vi "TLB Native Dynamic Events ver 0.17.vi"() -> ()   [LabVIEW 2018]
uses:
  Labview Training Phase 2/Enum Controls/States for Action Engine.ctl
  TLB Type Definitions/State Type Definitions.ctl
  TLB Type Definitions/Intruction Type Definitions.ctl
  TLB Type Definitions/Encoder cluster.ctl
  TLB Type Definitions/PING CLUSTER.ctl
  <vilib>/Studica/Studica Toolkit/NavX/NavX.lvlib
  <vilib>/Studica/Studica Toolkit/Background/DIO Channel.ctl
  Underlying VI's/NavX VI/navX type def.ctl
  <vilib>/myRIO/Instrument Drivers/Utilities/Utilities.lvlib
  <vilib>/Studica/Studica Toolkit/Background/I2C Channel.ctl
  TLB Type Definitions/Vision cluster.ctl
  <vilib>/NI_Real-Time Target Support.lvlib
  TLB Type Definitions/Stepper cluster.ctl
  Experimental VI's/Archived VI's/MOTOR CONTROL NO PID Type Def.ctl
  Underlying VI's/I2C Master VI/I2C MASTER Type Def.ctl
  Underlying VI's/I2C Master VI/I2C_MASTER_WRITE_NEW Type Def.ctl
  <vilib>/userdefined/High Color/IMAQdx.ctl
  Underlying VI's/I2C Master VI/Arduino_Interfacing.ctl
  TLB Type Definitions/Yaw Cluster.ctl
  TLB Type Definitions/Time cluster.ctl
  TLB Type Definitions/Y Stepper cluster.ctl
  Underlying VI's/Modified webcam FGV/Webcam AE.ctl
  Underlying VI's/Elasped Timer/Elapsed timer control.ctl
  Underlying VI's/Motor Control VI with PID/MOTOR CONTROL WITH PID AE DATA MODE TYPE DEF.ctl
  Underlying VI's/Motor Control VI with PID/MOTOR CONTROL WITH PID AE DIRECTION TYPE DEF.ctl
  TLB Type Definitions/IR Sensor Type Def.ctl
  <vilib>/myRIO/Common/Instrument Driver Framework/myRIO v1.0/AI/typedefs/AI Channels Enum.ctl
  <vilib>/myRIO/Common/Instrument Driver Framework/myRIO v1.0/AI/typedefs/AI Channels List.ctl
  <vilib>/Utility/RT CPU Load.ctl
panel:
  out "Left IR Sensor":dbl
  out "Obstacle detected":bool
  out "Speed & distance":T1
  out "Object Center Coordinates":cluster{"x":sgl, "y":sgl}
  out "Object detection cluster":T2
  out "Time up flag":bool
  out "Task selection":u8
  in  "Object recognition mode":enum16{"Ball", "Soap", "Gel", "Pipe", "None"}(ring)
  out "NavX Readings":T3
  out "Arduino Data":T4
  out "CPU loads":T5[](array[typedef]) {"ISR (%)" format="%#.2f"; "Idle (%)" format="%#.2f"; "Background (%)" format="%#.2f"; "Normal (%)" format="%#.2f"; "Above Normal (%)" format="%#.2f"; "High (%)" format="%#.2g"; "Timed Structures (%)" format="%#.2g"; "Time Critical (%)" format="%#.2g"; "Total (%)" format="%#.2g"}
  out "TASK ENABLE":bool
  out "Rising Edge":bool
  in  "Green LED":bool
  out "I2C Error":errorcluster
  out "State Logic":T6=enum."Startup"
  out "elements":T7[](array[typedef])
  in  "STOP TASK":bool
  in  "OK Button":bool
  in  "STOP":bool
  out "error out":errorcluster
  out "Action Queue Items":i32
  out "State Logic Queue Items":i32
  out "Action Queues items":string[](array[string])=["Hardware reset", "Software reset", ""]
  out "Action State":string
  # "System Health Status Update"
  # "VISION"
  # "TLB FRAMEWORK STATUS"
  # "Test Programme written by Calvin Loke    Dated: 28 Aug 2019\nTest Programme revised by Dr Alex See   Dated 30 Aug 2019\n\nRevision date: 20/03/2020\nProgramme version:   TLB Native Dynamic Events ver 0.14a"
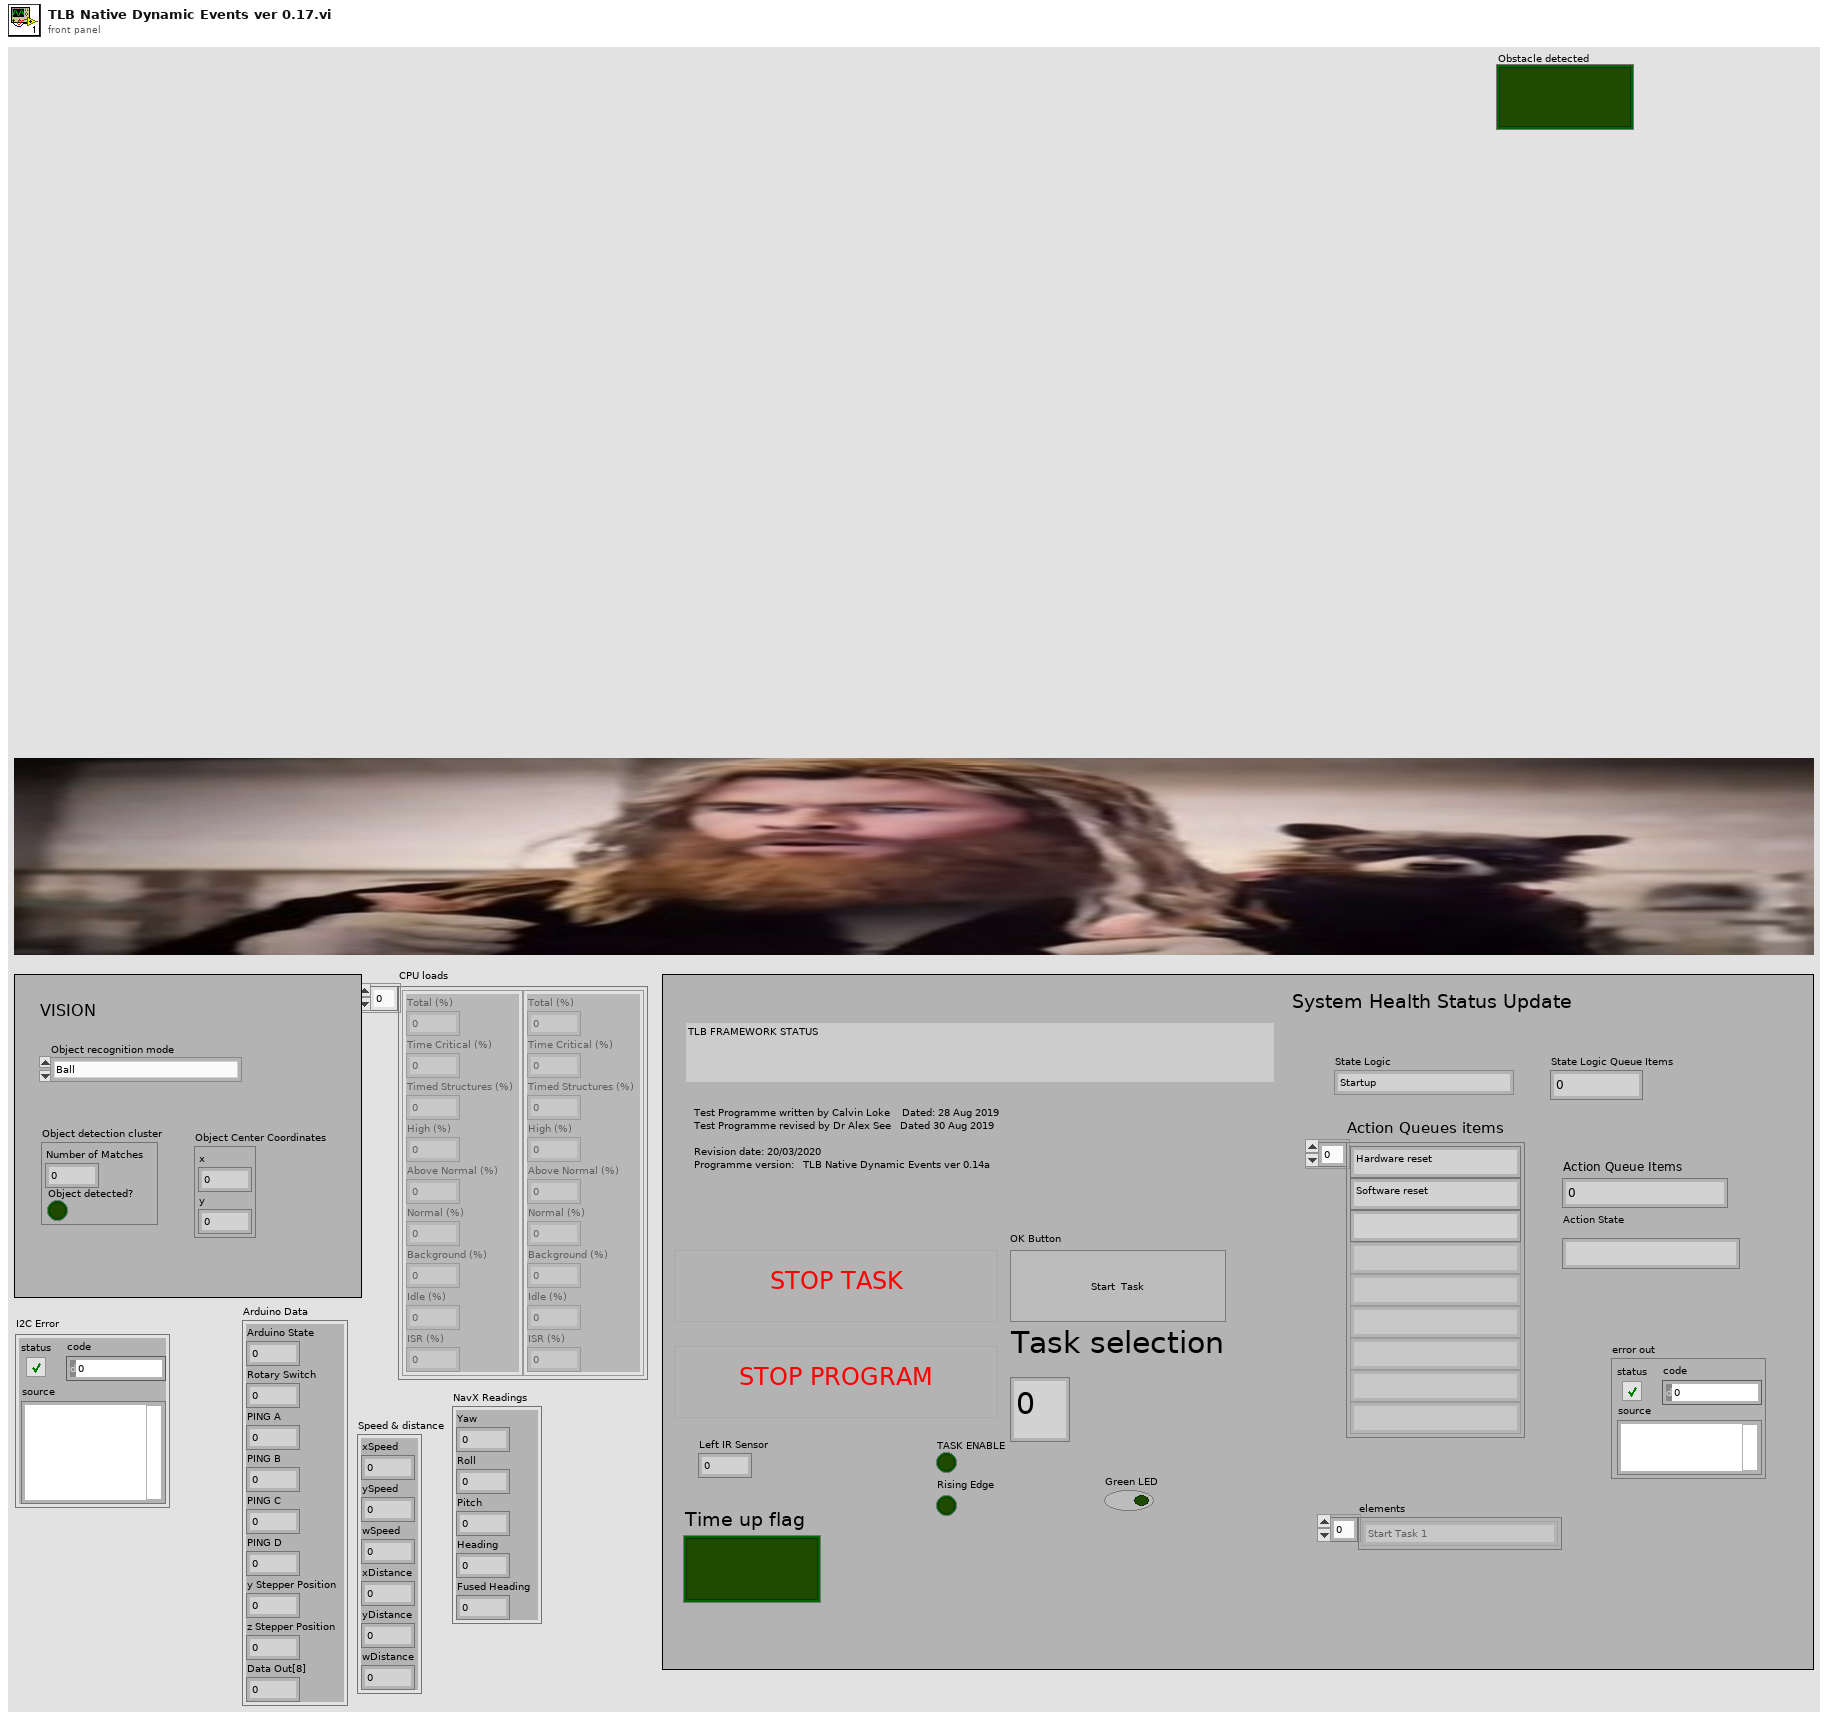
[diagram p1: front panel]
types:
  T1 = cluster{"xSpeed":dbl, "ySpeed":dbl, "wSpeed":dbl, "xDistance":dbl, "yDistance":dbl, "wDistance":dbl}
  T2 = cluster{"Number of Matches":i32, "Object detected?":bool}
  T3 = cluster{"Yaw":dbl, "Roll":dbl, "Pitch":dbl, "Heading":dbl, "Fused Heading":dbl}
  T4 = cluster{"Arduino State":u8, "Rotary Switch":u8, "PING A":u8, "PING B":u8, "PING C":u8, "PING D":u8, "y Stepper Position":u8, "z Stepper Position":u8, "Data Out[8]":u8}
  T5 = typedef "NI_Real-Time Target Support.lvlib/RT CPU Load.ctl" = cluster{"Total (%)":dbl, "Time Critical (%)":dbl, "Timed Structures (%)":dbl, "High (%)":dbl, "Above Normal (%)":dbl, "Normal (%)":dbl, "Background (%)":dbl, "Idle (%)":dbl, "ISR (%)":dbl}
  T6 = typedef "State Type Definitions.ctl" = enum16{"None", "Startup", "Move to Angle", "True Stop", "Idle", "Shutdown", "Task 1A", "Task 1B", "Task 2:Raise Arm", "Task 2:Sensor Mode", "Task 2:Reverse Mode", "Task 3", "Task 4_A", "Task 4_B", "Task 4_C", "Task 4_D", "Task 5A", "Task 5B", "Task 5C", "Task 5D", "Task 5E: POSITION ARM", "Task 5F: ARM GRAB HEIGHT", "Task 5G: CLOSE CLAW", "Task 5H: RAISE ARM", "Task 6_A", "Task 6_B", "Task 7", "Task 8A: RAISE ARM", "Task 8B: MOVE TO BOX", "Task 8C: CAM BURST", "Task 8D: PROCESS IMAGE", "Task 8E: ROBOT ADJUST", "Task 8F: CAM BURST 2", "Task 8G: PROCESS IMAGE 2", "Task 8H: ARM ADJUST", "Task 8I: ARM GRAB HEIGHT", "Task 8J: CLOSE CLAW", "Task 8K: RAISE MY SWORD", "Task 9A: Raise Arm", "Task 9B: Rotate to Angle", "Task 9C: Detect Box", "Task 9D: MOVE FORWARD", "Task 9E: MOVE LEFT", "Task 9F: SCAN IMAGE", "Task 9G: PROCESS COLOUR", "Task 9H: MOVE RIGHT", "Task 9I: SCAN IMAGE", "Task 9J: PROCESS COLOUR", "Task 9K: ROTATE 90 CW", "Task 9L: MOVE FORWARD", "Task 9M: MOVE RIGHT", "Task 9N: SCAN IMAGE", "Task 9O: PROCESS COLOUR", "Task 9P: MOVE RIGHT", "Task 9Q: SCAN IMAGE", "Task 9R: PROCESS COLOUR", "Task A1: Raise Arm", "Task A2: Rotate to Angle", "Task A3: Move Forward", "Task A4: Rotate CW 90"}
  T7 = typedef "Intruction Type Definitions.ctl" = enum16{"None", "Start Task 1", "Start Task 2", "Start Task 3", "Start Task 4", "Start Task 5", "Start Task 6", "Start Task 7", "Start Task 8 - BALL", "Start Task 8 - Gel", "Start Task 8 - Pipe", "Start Task 8 - Soap", "Start Task 9", "Start Task A", "Start Task B", "Exit"}
  T8 = typedef "IR Sensor Type Def.ctl" = cluster{"Left IR Sensor":dbl, "Arm IR Sensor":dbl, "Bottom IR Sensor":dbl}
  T9 = typedef "Y Stepper cluster.ctl" = cluster{"yStepper desired":u8}
  T10 = typedef "Time cluster.ctl" = cluster{"Time up flag":bool, "SET TIME TO CHECK":dbl}
  T11 = typedef "Yaw Cluster.ctl" = cluster{"Yaw":dbl, "Compass":dbl}
  T12 = typedef "Stepper cluster.ctl" = cluster{"y Stepper Position":u8, "z Stepper Position":u8}
  T13 = typedef "DIO Channel.ctl" = enum16{"Not Connected", "A/DIO1", "A/DIO2", "A/DIO3", "A/DIO4", "A/DIO5", "A/DIO6", "A/DIO7", "A/DIO13", "B/DIO1", "B/DIO2", "B/DIO3", "B/DIO4", "B/DIO5", "B/DIO6", "B/DIO7", "B/DIO13", "C/DIO0", "C/DIO1", "C/DIO2", "C/DIO3", "C/DIO4", "C/DIO5", "C/DIO6", "C/DIO7"}
  T14 = typedef "Vision cluster.ctl" = cluster{"Recognized Object":bool, "Object X coordinate":dbl, "Object Y coordinate":dbl}
  T15 = typedef "PING CLUSTER.ctl" = cluster{"PING_A":u8, "PING_B":u8, "PING_C":u8, "PING_D":u8}
  T16 = typedef "Encoder cluster.ctl" = cluster{"xDistance":dbl, "yDistance":dbl, "wDistance":dbl}
  T17 = cluster{"DIO Channel":T13, "FPGA VI Reference Out":refnum<k20>}
  T18 = typedef "navX type def.ctl" = enum16{"Get i2C reference", "Read Values", "Zero Yaw"}
  T19 = typedef "Arduino_Interfacing.ctl" = enum16{"Initialize", "Write to Arduino", "Read From Arduino"}
  T20 = typedef "I2C Channel.ctl" = enum16{"Not Connected", "A", "B"}
  T21 = typedef "States for Action Engine.ctl" = enum16{"Initialize", "Write", "Read"}
  T22 = cluster{"I2C Ref Out":cluster{"I2C Channel":T20, "FPGA VI Reference Out":refnum<k20>}, "Connected":bool, "Slave Address (7-bit)":u8, "Registry":u8[]}
  T23 = typedef "IMAQ Image.ctl" = refnum<image>
  T24 = typedef "State Type Definitions.ctl" = enum16{"None", "Startup", "Move to Angle", "True Stop", "Idle", "Shutdown", "Task 1", "Task 2:Raise Arm", "Task 2:Sensor Mode", "Task 3", "Task 4_A", "Task 4_B", "Task 4_C", "Task 4_D", "Task 5_A", "Task 5 _B", "Task 5_C", "Task 5_D", "Task 5_D_Error", "Task 5D_Error_Right", "Task 5D_Error_Left", "Task 5_E", "Task 5_F", "Task 5F_Error", "Task 5G", "Task 5H", "Task 5I", "Task 6_A", "Task 6_B", "Task 7", "Task 8", "Task 9A: Raise Arm", "Task 9B: Rotate to Angle", "Task 9C: Rotation alignmnet", "Task B"}
  T25 = typedef "MOTOR CONTROL WITH PID AE DIRECTION TYPE DEF.ctl" = enum16{"y-axis movement", "x-axis movement", "rotation", "stop", "reset encoders"}
  T26 = typedef "MOTOR CONTROL WITH PID AE DATA MODE TYPE DEF.ctl" = enum16{"Init AE", "Write to AE", "Read from AE"}
  T27 = typedef "Elapsed timer control.ctl" = enum16{"Start", "Pause", "Initialize"}
  T28 = typedef "I2C_MASTER_WRITE_NEW Type Def.ctl" = enum16{"Ultrasonic sensors", "Stepper origin", "zStepper 13.3k", "zStepper 13k", "zStepper 12k", "zStepper 11k", "zStepper 10k", "zStepper 9k", "zStepper 8k", "zStepper 7k", "zStepper 6k", "zStepper 5k", "zStepper 4k", "zStepper 3k", "zStepper 2k", "zStepper 1k", "zStepper 900", "zStepper 800", "zStepper 700", "zStepper 600", "zStepper 500", "zStepper 400", "zStepper 300", "zStepper 200", "zStepper 100", "zStepper 0", "yStepper control", "Open Claw", "Close Claw", "Soft Reset"}
  T29 = typedef "Webcam AE.ctl" = enum16{"Initialize Camera", "Open Camera", "Continuous Acquisition", "Close Camera", "Retrieve Image", "Dispose Camera Image Buffer"}
  T30 = typedef "IMAQdx.ctl" = refnum<k21>
  T31 = typedef "Webcam AE.ctl" = enum16{"Initialize Camera", "Open Camera", "Continuous Acquisition", "Close Camera", "Retrieve Image", "Dispose Image Buffers"}
  T32 = typedef "MOTOR CONTROL NO PID Type Def.ctl" = enum16{"Init", "Front Back", "Left Right", "Rotate", "Stop", "Latch"}
  T33 = typedef "AI Channels List.ctl" = T34[]
  T34 = typedef "AI Channels Enum.ctl" = enum16{"Not Connected", "AudioIn/Left", "AudioIn/Right", "C/AI0", "C/AI1", "A/AI0", "A/AI1", "A/AI2", "A/AI3", "A/AI4", "A/AI5", "A/AI6", "A/AI7", "B/AI0", "B/AI1", "B/AI2", "B/AI3", "B/AI4", "B/AI5", "B/AI6", "B/AI7", "AI/AI0", "AI/AI1", "AI/AI2", "AI/AI3", "A/AI0 (DIFF)", "A/AI1 (DIFF)", "A/AI2 (DIFF)", "A/AI3 (DIFF)", "B/AI0 (DIFF)", "B/AI1 (DIFF)", "B/AI2 (DIFF)", "B/AI3 (DIFF)"}
  T35 = typedef "I2C MASTER Type Def.ctl" = enum16{"Last State", "Mode 0", "Mode 1", "Mode 2", "Mode 3", "Mode 4", "Mode 5", "Mode 6", "Mode 7", "Mode 8", "Mode 9", "Mode 10"}
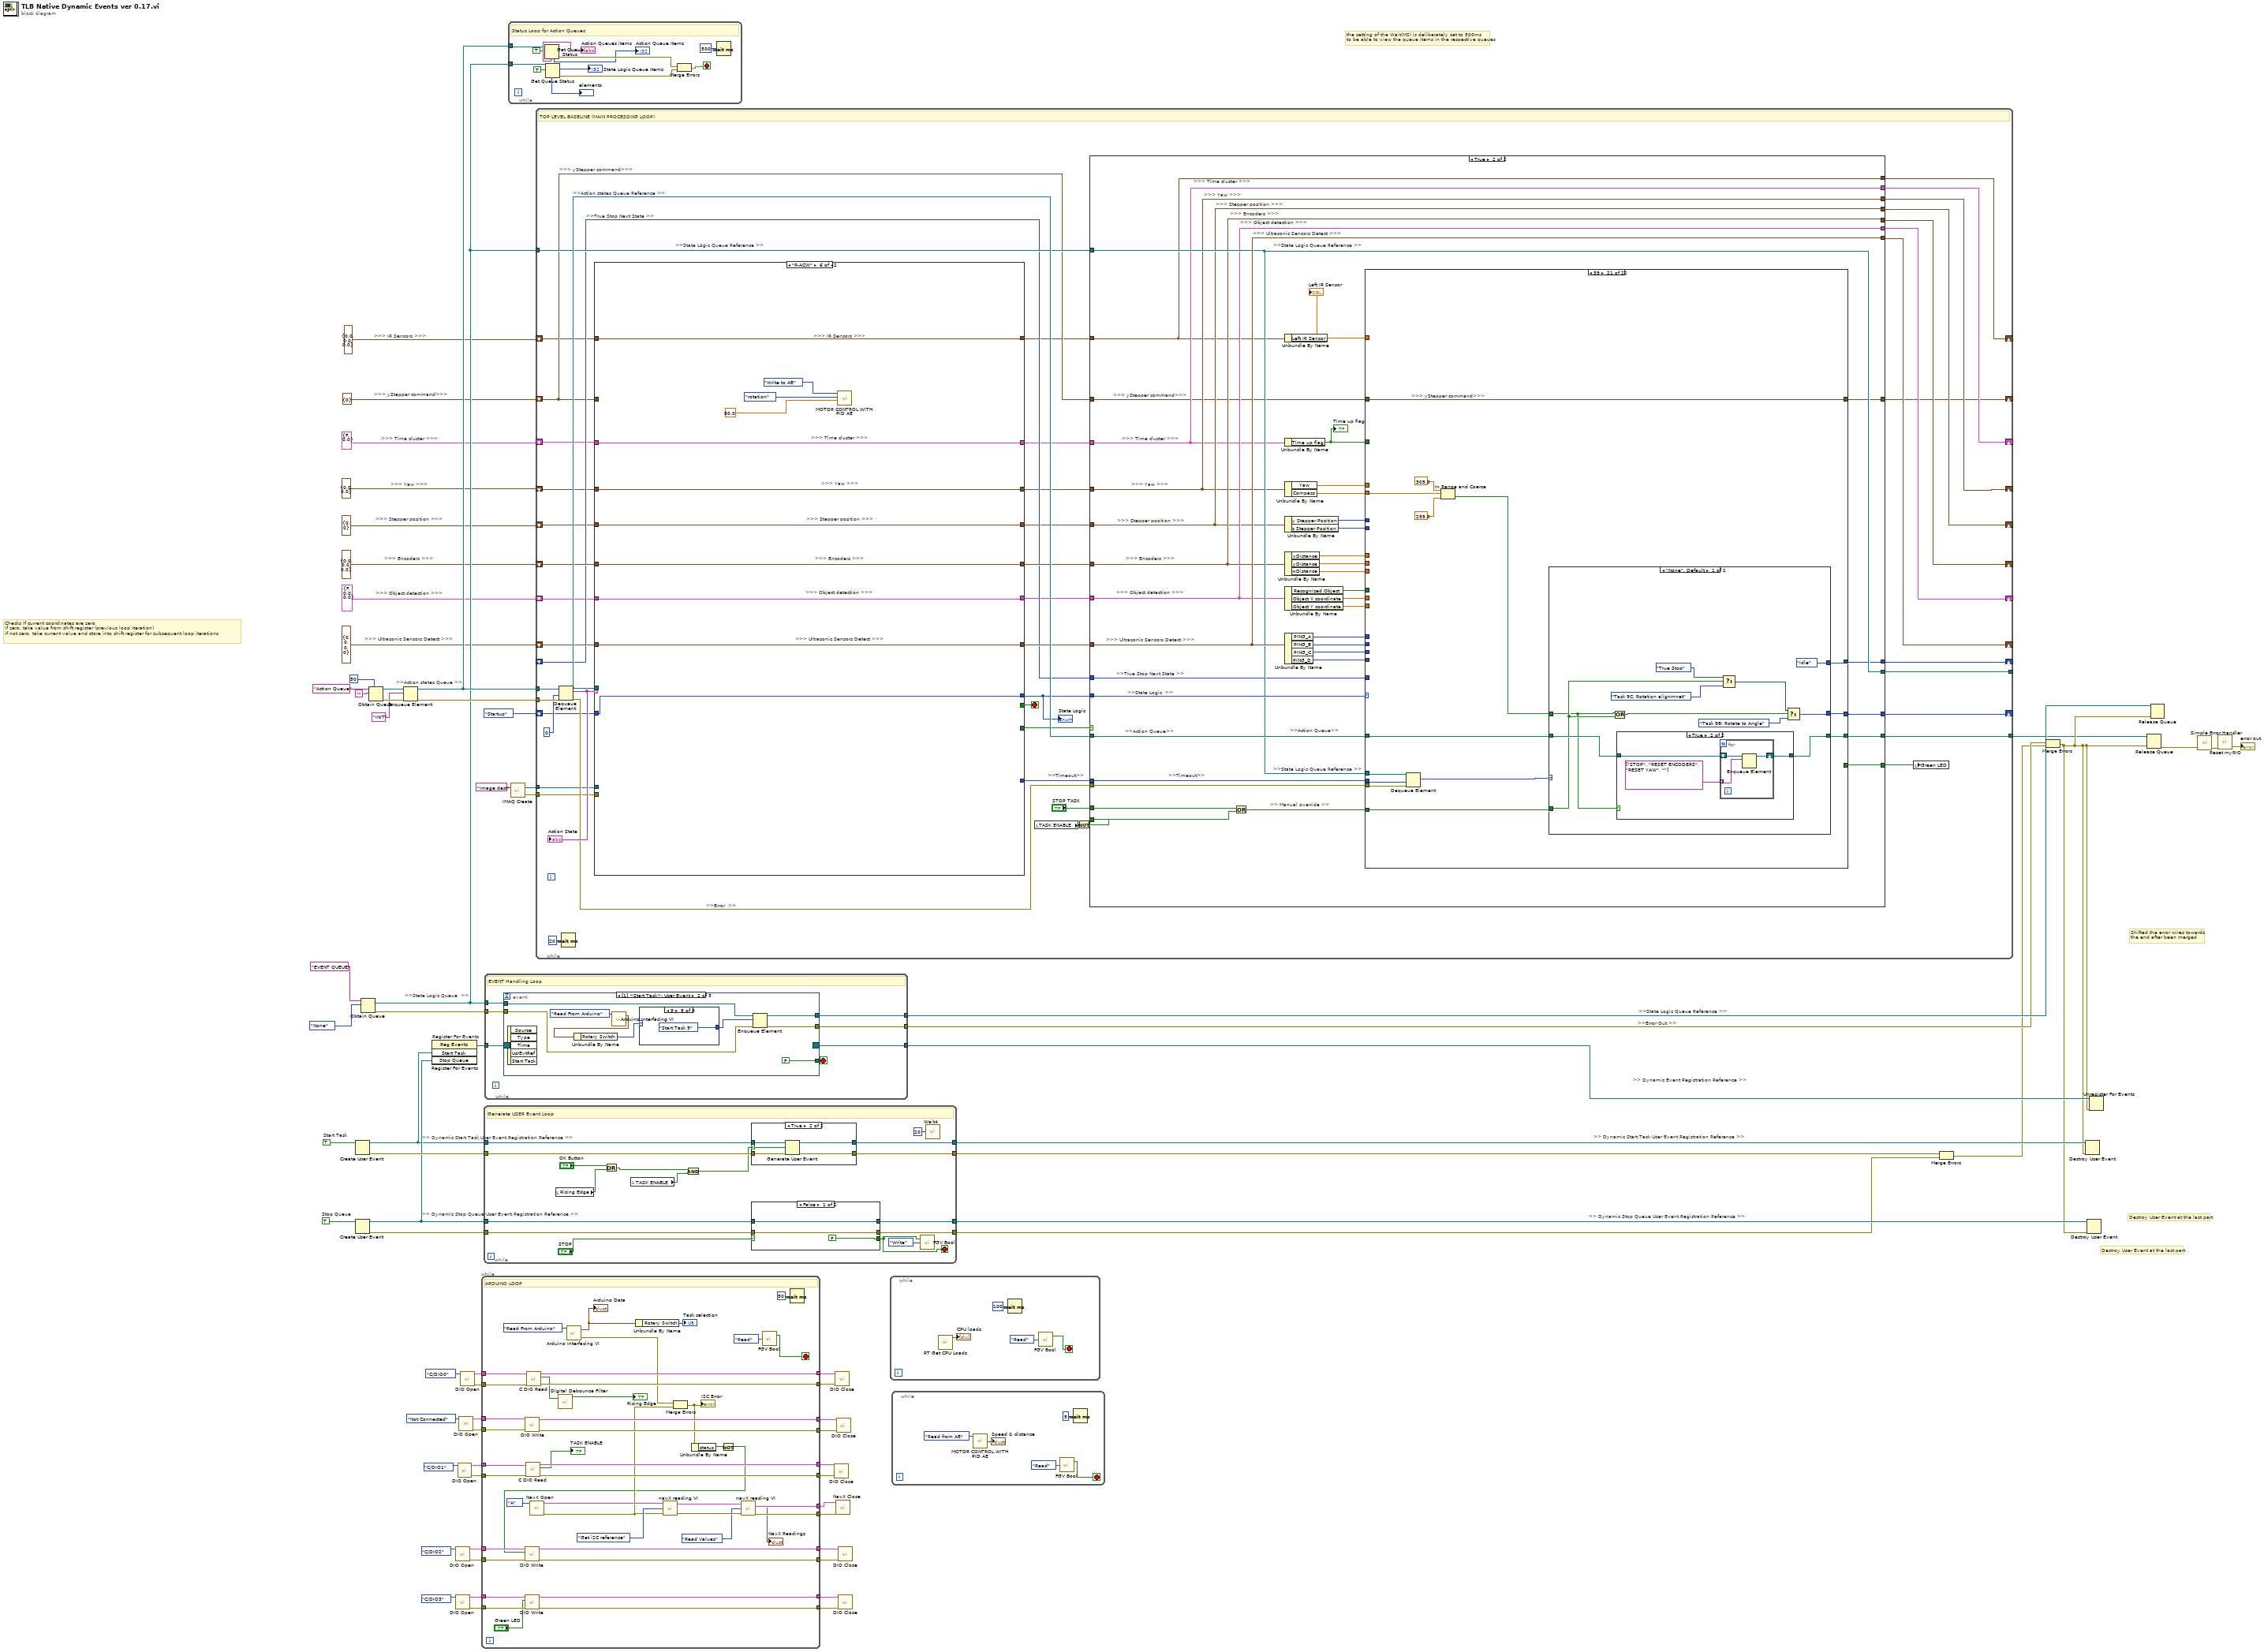
[diagram p0: block diagram]
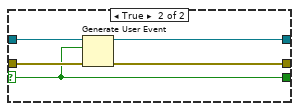
[diagram p2: hidden frame]
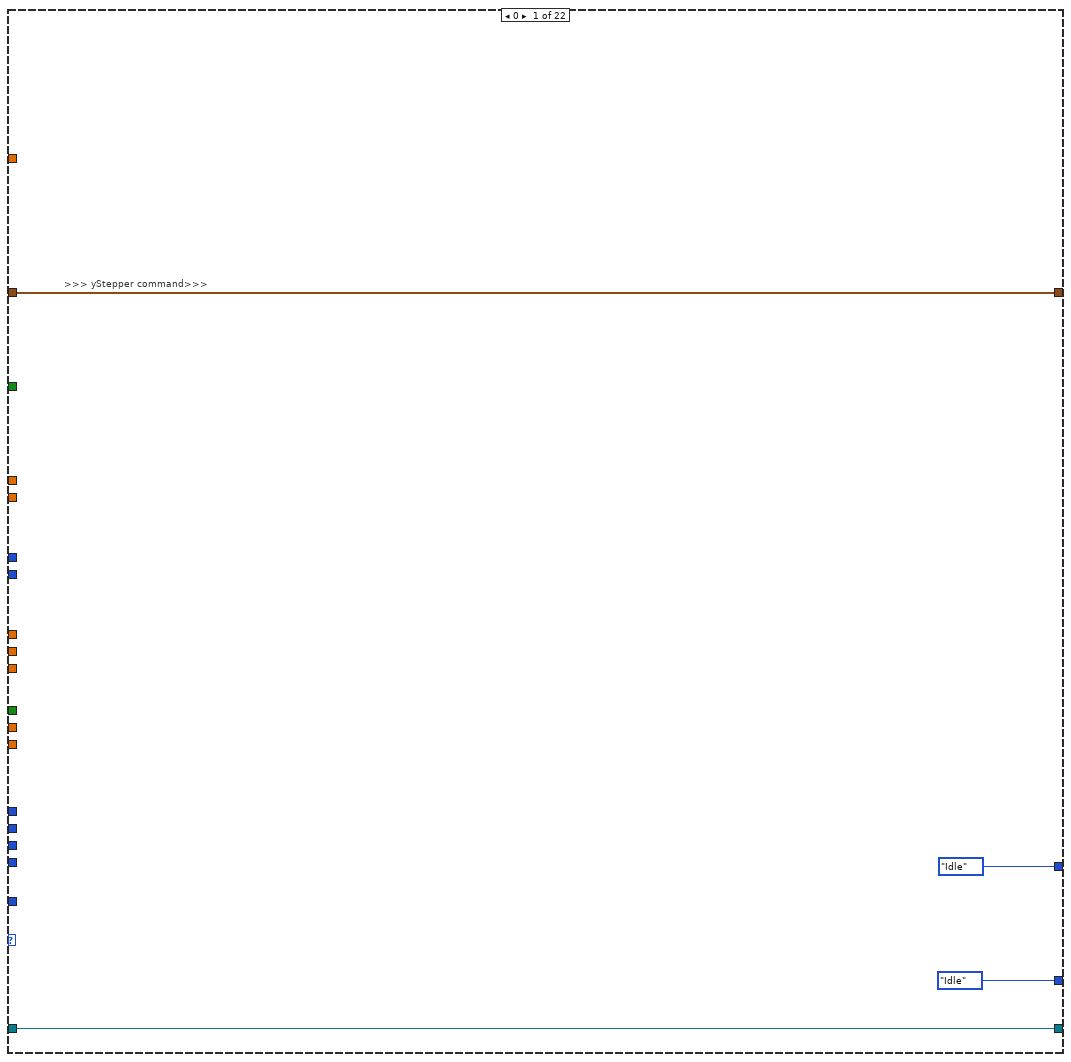
[diagram p5: hidden frame]
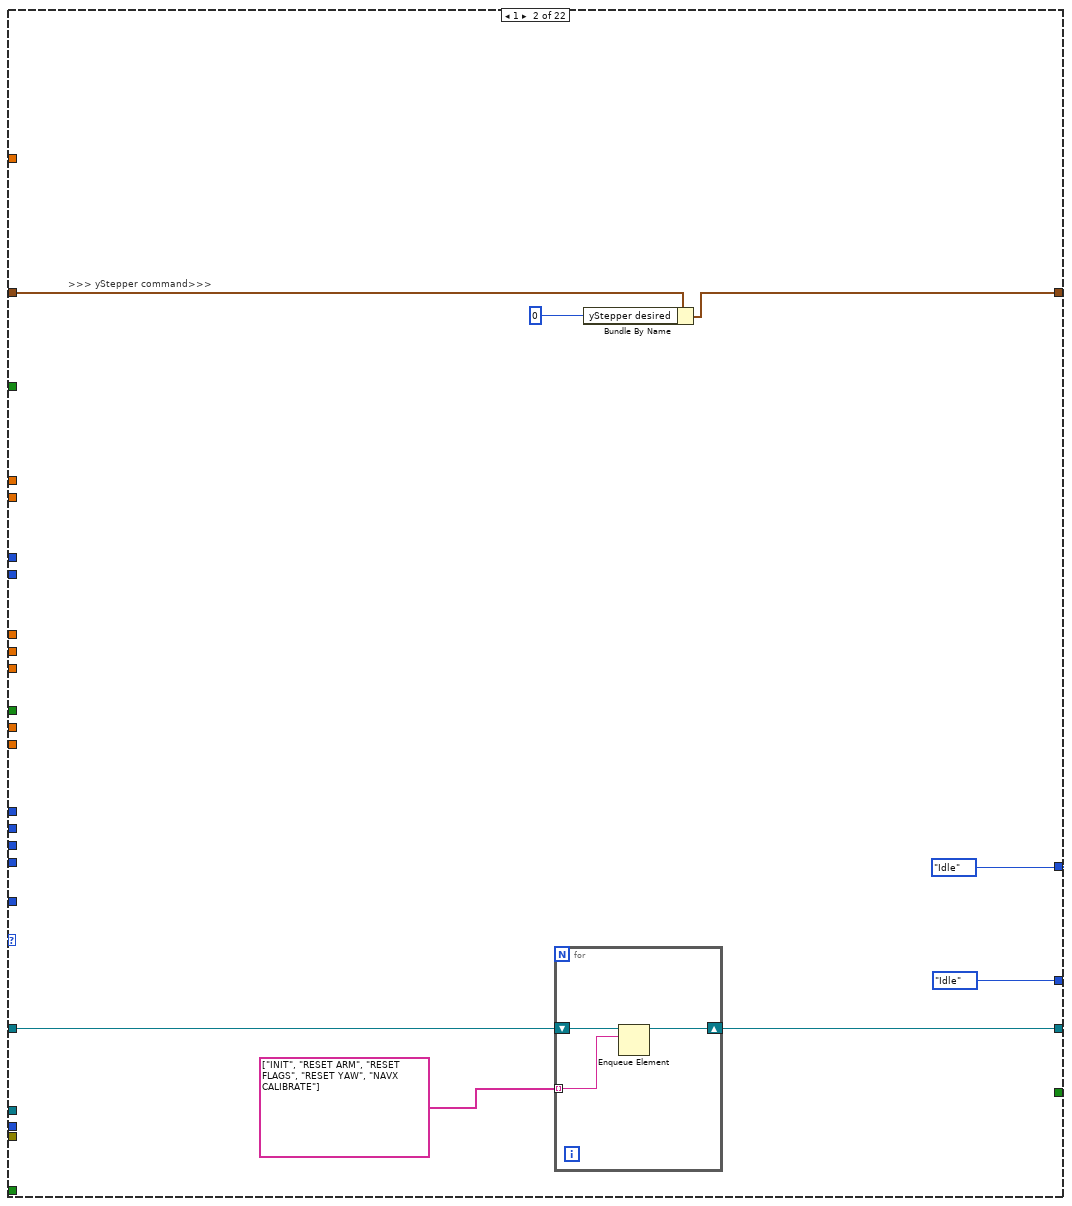
[diagram p6: hidden frame]
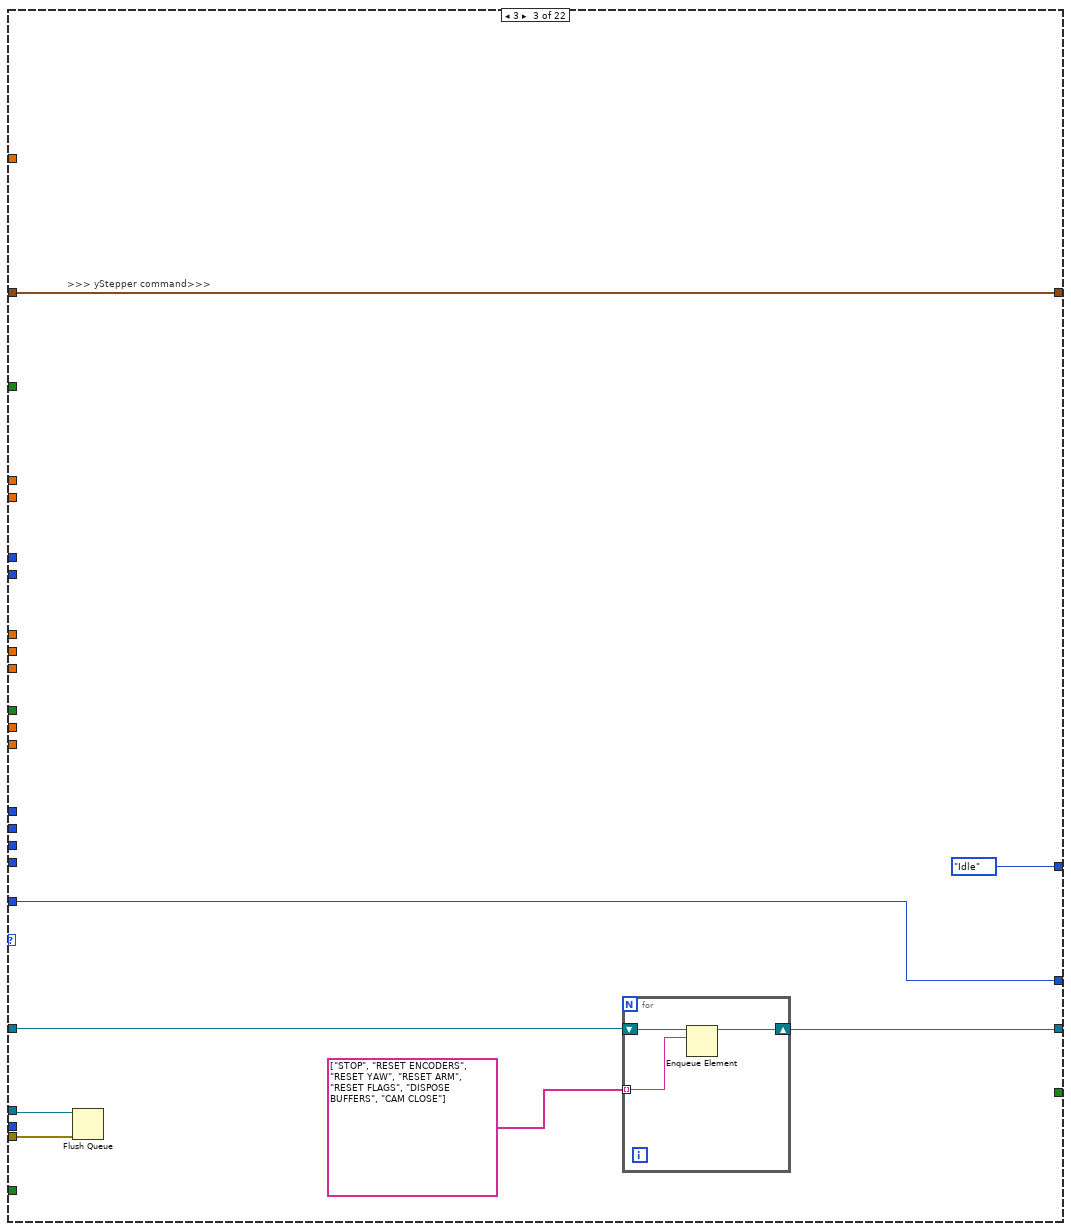
[diagram p7: hidden frame]
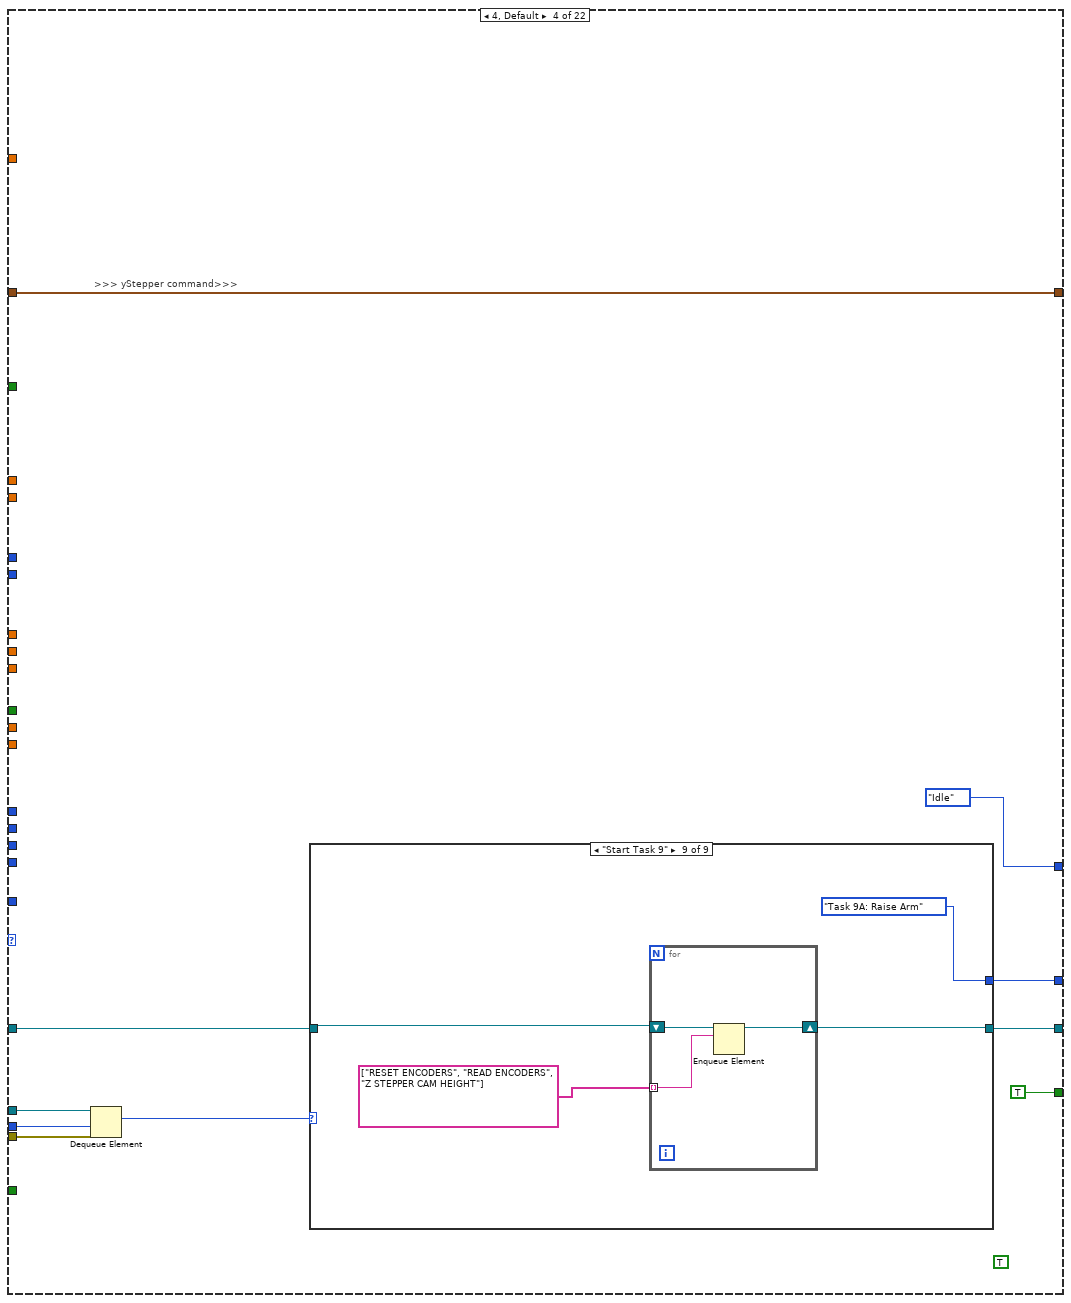
[diagram p8: hidden frame]
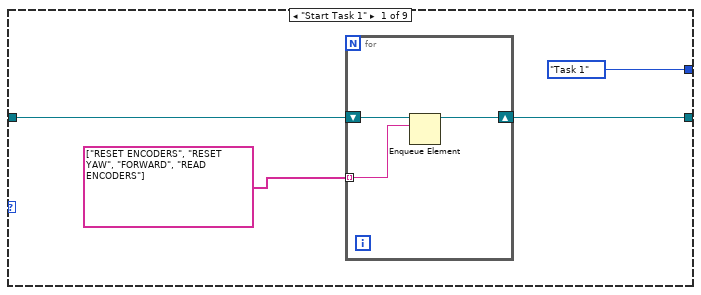
[diagram p9: hidden frame]
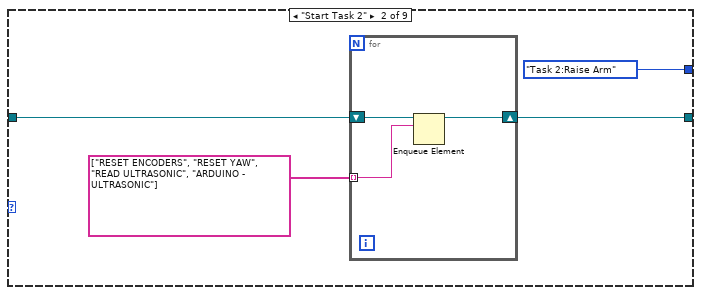
[diagram p10: hidden frame]
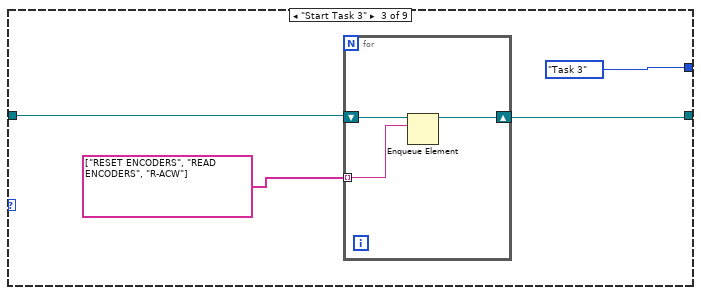
[diagram p11: hidden frame]
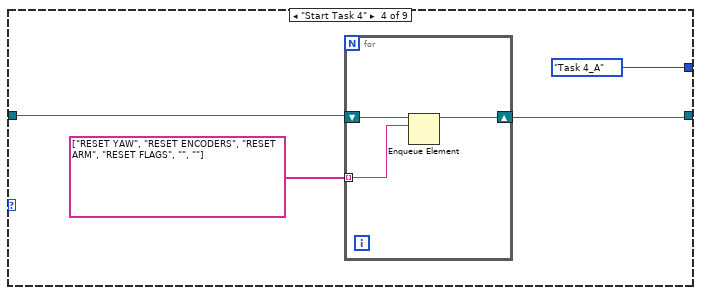
[diagram p12: hidden frame]
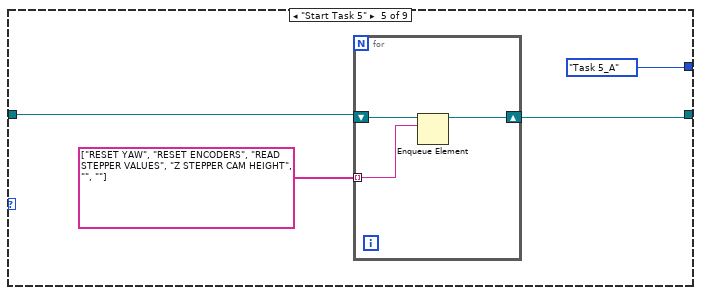
[diagram p13: hidden frame]
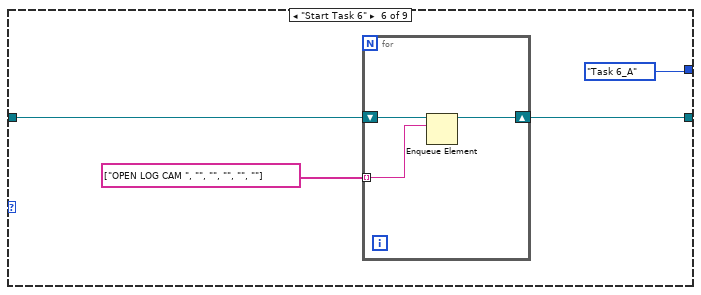
[diagram p14: hidden frame]
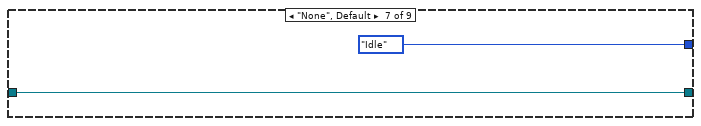
[diagram p15: hidden frame]
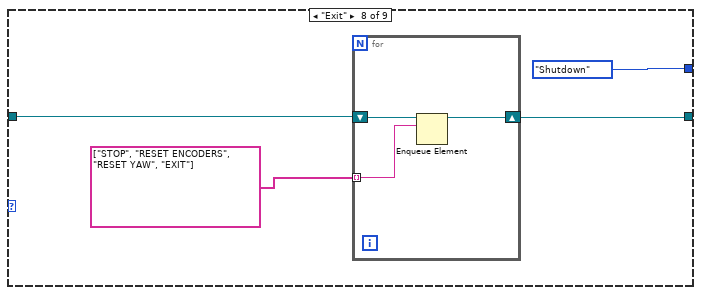
[diagram p16: hidden frame]
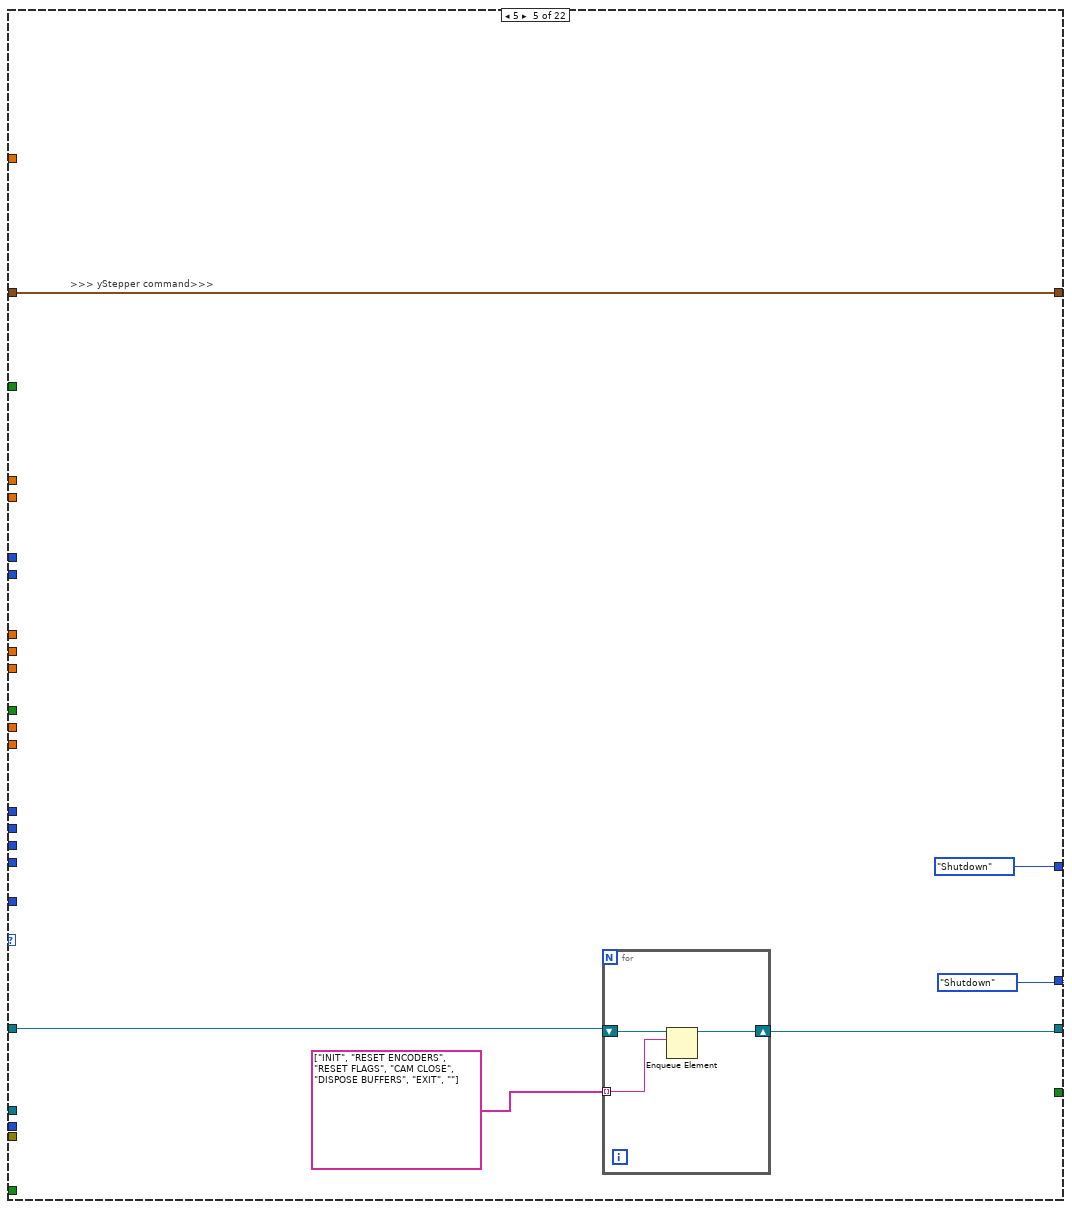
[diagram p17: hidden frame]
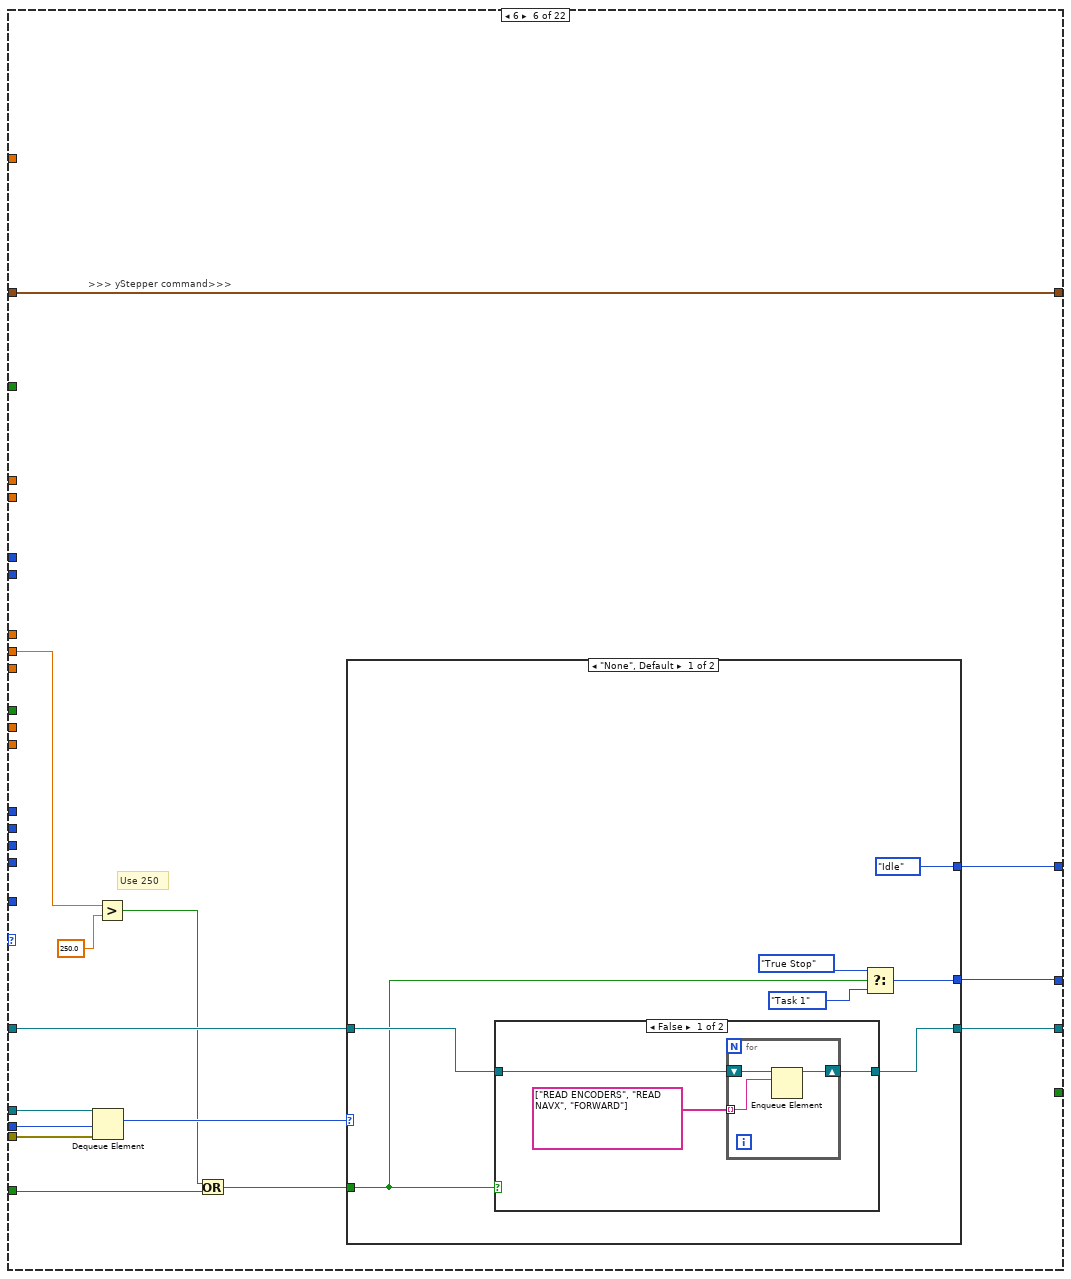
[diagram p18: hidden frame]
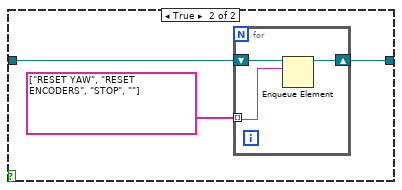
[diagram p19: hidden frame]
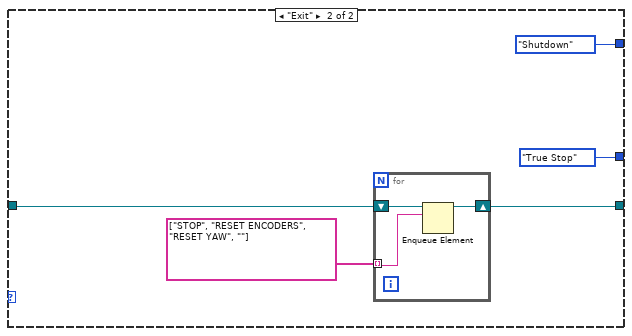
[diagram p20: hidden frame]
diagram:
  w71 = TRUE  # Stop Queue
  w70 = TRUE  # Start Task
  # ">>> IR Sensors >>>"
  # "Checks if current coordinates are zero\nif zero, take value from shift register (previous loop iteration)\nif not zero, take current value and store into shift register for subsequent loop iterations"
  # ">>> yStepper command>>>"
  # ">>> Time cluster >>>"
  # ">>> Yaw >>>"
  # ">>> Stepper position >>>"
  # ">>> Encoders >>>"
  # ">>> Object detection >>>"
  # ">>> Ultrasonic Sensors Detect >>>"
  # "the setting of the Wait(MS) is deliberately set to 500ms\nto be able to view the queue items in the respective queues"
  # ">>Error Out >>"
  # ">> Dynamic Stop Queue User Event Registration Reference >>"
  # ">> Dynamic Start Task User Event Registration Reference >>"
  # ">> Dynamic Stop Queue User Event Registration Reference >>"
  # ">> Dynamic Start Task User Event Registration Reference >>"
  # ">> Dynamic Event Registration Reference >>"
  # ">>Action states Queue >>"
  # ">>State Logic Queue  >>"
  # ">>State Logic Queue Reference >>"
  # "Destroy User Event at the last part"
  # "Destroy User Event at the last part"
  # "Shifted the error wires towards\nthe end after been merged"
  n1 = Create User Event(user event datatype=w70) -> (user event=w62:refnum<user-event>, error out=w67:errorcluster)  [unwired: 1 in]
  n2 = Create User Event(user event datatype=w71) -> (user event=w63:refnum<user-event>, error out=w66:errorcluster)  [unwired: 1 in]
  n3 = Obtain Queue(name (unnamed)="EVENT QUEUE", element data type=Intruction_Type_Definitions."None" ("Enum")) -> (queue out=w48:refnum<queue>, error out=w54:errorcluster)  [unwired: 3 in, 1 out]
  n4 = Obtain Queue(max queue size (-1, unlimited)=50, name (unnamed)="Action Queue", element data type="") -> (queue out=w57:refnum<queue>, error out=w53:errorcluster)  [unwired: 2 in, 1 out]
  n5 = Enqueue Element(queue=w57, element="INIT", error in (no error)=w53) -> (queue out=w49:refnum<queue>, error out=w52:errorcluster)  [unwired: 1 in, 1 out]
  n6 = register-events "Register For Events"(w62, w63) -> (reference out=w61:refnum<event-registration>)  [unwired: 2 in, 1 out]
  n7 = call <vilib>:"DIO Open.vi"("DIO Channel"=DIO_Channel."C/DIO2") -> ("error out"=w15:errorcluster, "DIO Info Out"=w16:T17)  [unwired: 9 in]
  n8 = call <vilib>:"DIO Open.vi"("DIO Channel"=DIO_Channel."C/DIO3") -> ("error out"=w10:errorcluster, "DIO Info Out"=w11:T17)  [unwired: 9 in]
  n9 = call <vilib>:"DIO Open.vi"("DIO Channel"=DIO_Channel."C/DIO1") -> ("error out"=w26:errorcluster, "DIO Info Out"=w27:T17)  [unwired: 9 in]
  n10 = call <vilib>:"DIO Open.vi"("DIO Channel"=DIO_Channel."Not Connected") -> ("error out"=w31:errorcluster, "DIO Info Out"=w33:T17)  [unwired: 9 in]
  n11 = call <vilib>:"DIO Open.vi"("DIO Channel"=DIO_Channel."C/DIO0") -> ("error out"=w36:errorcluster, "DIO Info Out"=w39:T17)  [unwired: 9 in]
  n12 = while {
    tunnel: w39 -> [w112]
    tunnel: [w111] -> w37
    tunnel: w36 -> [w110]
    tunnel: [w109] -> w35
    tunnel: w33 -> [w106]
    tunnel: [w105] -> w32
    tunnel: w31 -> [w104]
    tunnel: [w103] -> w30
    tunnel: [w102] -> w28
    tunnel: w27 -> [w101]
    tunnel: w26 -> [w100]
    tunnel: [w99] -> w25
    tunnel: w16 -> [w93]
    tunnel: w15 -> [w92]
    tunnel: [w91] -> w14
    tunnel: [w90] -> w13
    tunnel: w11 -> [w89]
    tunnel: w10 -> [w88]
    tunnel: [w87] -> w9
    tunnel: [w86] -> w8
    tunnel: [w80] -> w5
    tunnel: [w79] -> w6
    stop <- w114 stop-if-true
    # "ARDUINO LOOP"
    n13 = call <vilib>:"DIO Write.vi"("error in (no error)"=w88, "Input"="Green LED", "DIO Info In"=w89) -> ("error out"=w86:errorcluster, "DIO Info Out"=w87:T17)  [unwired: 7 in]
    n14 = call <vilib>:"DIO Write.vi"("error in (no error)"=w104, "DIO Info In"=w106) -> ("error out"=w103:errorcluster, "DIO Info Out"=w105:T17)  [unwired: 8 in]
    n15 = call <vilib>:"C DIO Read.vi"("error in (no error)"=w100, "DIO Info In in"=w101) -> ("error out"=w99:errorcluster, "IN"=→"TASK ENABLE":bool, "DIO Info In out"=w102:T17)  [unwired: 7 in]
    n16 = call <vilib>:"C DIO Read.vi"("error in (no error)"=w110, "DIO Info In in"=w112) -> ("error out"=w109:errorcluster, "IN"=w108:bool, "DIO Info In out"=w111:T17)  [unwired: 7 in]
    n17 = call <vilib>:"NavX Open.vi"("I2C Channel"=I2C_Channel."A") -> ("error out"=w95:errorcluster, "NavX Info"=w97:T22)  [unwired: 9 in]
    n18 = call "Digital Debounce Filter.vi"("Boolean input"=w108) -> ("Rising Edge"=→"Rising Edge":bool)  [unwired: 1 in, 2 out]
    n19 = call "Arduino Interfacing VI.vi"("AE Mode"=Arduino_Interfacing."Read From Arduino") -> ("error out"=w83:errorcluster, "Arduino Data"=w76:T4)  [unwired: 3 in]
    "Arduino Data" <- w76
    n20 = Unbundle By Name(w76) -> ("Rotary Switch"=→"Task selection":u8)
    n21 = call "navX reading VI.vi"("NavX Info In"=w97, "Mode"=navX_type_def."Get i2C reference", "error in (no error)"=w95) -> ("NavX Info Out"=w82:T22, "Error Out"=w81:errorcluster)  [unwired: 2 out]
    n22 = Merge Errors(w83, w95) -> (w74:errorcluster)
    "I2C Error" <- w74
    n23 = Unbundle By Name(w74) -> ("status"=w73:bool)
    n24 = Not(x=w73) -> (.not. x?=w72:bool)
    n25 = call <vilib>:"DIO Write.vi"("error in (no error)"=w92, "Input"=w72, "DIO Info In"=w93) -> ("error out"=w90:errorcluster, "DIO Info Out"=w91:T17)  [unwired: 7 in]
    n26 = call "navX reading VI.vi"("NavX Info In"=w82, "Mode"=navX_type_def."Read Values", "error in (no error)"=w81) -> ("NavX Info Out"=w80:T22, "NavX Readings"=→"NavX Readings":T3, "Error Out"=w79:errorcluster)  [unwired: 1 out]
    n27 = call "FGV Bool.vi"("Init/Read/Write State"=States_for_Action_Engine."Read") -> ("Output node"=w114:bool)  [unwired: 2 in, 1 out]
    n28 = Wait (ms)(milliseconds to wait=u32 50) -> ()  [unwired: 1 out]
  }
  n29 = while {
    tunnel: w62 -> [w132]
    tunnel: w63 -> [w131]
    tunnel: [w130] -> w69
    tunnel: [w129] -> w68
    tunnel: w67 -> [w128]
    tunnel: [w127] -> w65
    tunnel: w66 -> [w126]
    tunnel: [w125] -> w64
    stop <- w123 stop-if-true
    # "Generate USER Event Loop"
    n30 = local read "Rising Edge"() -> (w119:bool)
    n31 = Or(x="OK Button", y=w119) -> (x .or. y?=w118:bool)
    n32 = local read "TASK ENABLE"() -> (w117:bool)
    n33 = And(x=w118, y=w117) -> (x .and. y?=w116:bool)
    n34 = case shown="True" w116 {
      selector: w116 -> [_ w143]
      tunnel: w132 -> [w142 w147]
      tunnel: [w142 w146] -> w129
      tunnel: w128 -> [w141 w145]
      tunnel: [w141 w144] -> w127
      frame False {
      }
      frame True {
        n35 = Generate User Event(user event=w147, event data cluster=w143, error in=w145) -> (user event out=w146:refnum<user-event>, error out=w144:errorcluster)  [unwired: 1 in]
      }
    }
    n36 = case shown="False" "STOP" {
      selector: "STOP" -> [_ w136]
      tunnel: w131 -> [w135 w140]
      tunnel: [w135 w139] -> w130
      tunnel: w126 -> [w134 w138]
      tunnel: [w134 w137] -> w125
      tunnel: [FALSE w136] -> w123
      frame False {
      }
      frame True {
        n37 = Generate User Event(user event=w140, event data cluster=w136, error in=w138) -> (user event out=w139:refnum<user-event>, error out=w137:errorcluster)  [unwired: 1 in]
      }
    }
    n38 = call "FGV Bool.vi"("Init/Read/Write State"=States_for_Action_Engine."Write", "Input Node"=w123) -> ()  [unwired: 1 in, 2 out]
    n39 = call "Wait4"("Count(uSec)"=u32 20) -> ()  [unwired: 1 out]
  }
  n40 = while {
    tunnel: w61 -> [w154]
    tunnel: [w153] -> w60
    tunnel: w48 -> [w151]
    tunnel: [w150] -> w59
    tunnel: w54 -> [w149]
    tunnel: [w148] -> w51
    stop <- w152 stop-if-true
    # "EVENT Handling Loop"
    n41 = event shown="[1] <Start Task>: User Event" {
      selector: w154 -> [_ _ _]
      dyn-events: [_ _ _] -> w153
      timeout: _ -> [_ _ _]
      tunnel: [FALSE FALSE w183] -> w152
      tunnel: w151 -> [w159 w168 w181]
      tunnel: [w158 w167 w182] -> w150
      tunnel: w149 -> [w157 w166 w180]
      tunnel: [w156 w165 w179] -> w148
      event Timeout {
        n42 = event-data() -> ()  [unwired: 1 in, 3 out]
        n43 = Enqueue Element(queue=w159, element=Intruction_Type_Definitions."None" ("Enum"), error in (no error)=w157) -> (queue out=w158:refnum<queue>, error out=w156:errorcluster)  [unwired: 1 in, 1 out]
      }
      event User Event {
        n44 = event-data() -> ()  [unwired: 1 in, 5 out]
        n45 = call "Arduino Interfacing VI.vi"("AE Mode"=Arduino_Interfacing."Read From Arduino") -> ("Arduino Data"=w162:T4)  [unwired: 3 in, 1 out]
        n46 = Unbundle By Name(w162) -> ("Rotary Switch"=w161:u8)
        n47 = case shown="9" w161 {
          tunnel: [Intruction_Type_Definitions."None" ("Enum") Intruction_Type_Definitions."Start Task 1" ("Enum") Intruction_Type_Definitions."Start Task 2" ("Enum") Intruction_Type_Definitions."Start Task 3" ("Enum") Intruction_Type_Definitions."Start Task 4" ("Enum") Intruction_Type_Definitions."Start Task 5" ("Enum") Intruction_Type_Definitions."Start Task 6" ("Enum") Intruction_Type_Definitions."Start Task 9" ("Enum")] -> w164
          frame 0, Default {
          }
          frame 1 {
          }
          frame 2 {
          }
          frame 3 {
          }
          frame 4 {
          }
          frame 5 {
          }
          frame 6 {
          }
          frame 9 {
          }
        }
        n48 = Enqueue Element(queue=w168, element=w164, error in (no error)=w166) -> (queue out=w167:refnum<queue>, error out=w165:errorcluster)  [unwired: 1 in, 1 out]
      }
      event User Event {
        n49 = event-data() -> ("Stop Queue"=w183:bool)  [unwired: 1 in, 4 out]
        n50 = Enqueue Element At Opposite End(queue=w181, element=Intruction_Type_Definitions."Exit" ("Enum"), error in (no error)=w180) -> (queue out=w182:refnum<queue>, error out=w179:errorcluster)  [unwired: 1 in, 1 out]
      }
    }
  }
  n51 = while {
    tunnel: w49 -> [w193]
    tunnel: w48 -> [w190]
    stop <- w187 stop-if-true
    # "Status Loop for Action Queues"
    n52 = Get Queue Status(queue=w193, return elements? (F)=TRUE) -> (error out=w189:errorcluster, # elements in queue=→"Action Queue Items":i32, elements=→"Action Queues items":string[])  [unwired: 1 in, 5 out]
    n53 = Get Queue Status(queue=w190, return elements? (F)=TRUE) -> (# pending remove=→"State Logic Queue Items":i32, error out=w188:errorcluster, elements=→"elements":T7[])  [unwired: 1 in, 5 out]
    n54 = Merge Errors(w189, w188) -> (w187:errorcluster)
    n55 = Wait (ms)(milliseconds to wait=u32 500) -> ()  [unwired: 1 out]
  }
  n56 = call "IMAQ Create"("Image Name"="Image dest") -> ("New Image"=w20:T23, "error out"=w19:errorcluster)  [unwired: 4 in]
  n57 = while {
    tunnel: w48 -> [w230]
    tunnel: w49 -> [w242]
    tunnel: w52 -> [w240]
    tunnel: [w239] -> _
    tunnel: [w238] -> w42
    shift-right: [w231] -> _
    shift-left: T15 {"PING_A"=0, "PING_B"=0, "PING_C"=0, "PING_D"=0} -> [w233]
    shift-right: [w224] -> _
    shift-left: State_Type_Definitions."Startup" ("Enum") -> [w227]
    shift-right: [w220] -> _
    shift-left: T16 {"xDistance"=0.0, "yDistance"=0.0, "wDistance"=0.0} -> [w222]
    shift-right: [w217] -> _
    shift-left: _ -> [w216]
    tunnel: w20 -> [w215]
    tunnel: w19 -> [w214]
    shift-right: [w211] -> _
    shift-left: T14 {"Recognized Object"=FALSE, "Object X coordinate"=0.0, "Object Y coordinate"=0.0} -> [w213]
    shift-right: [w208] -> _
    shift-left: T12 {"y Stepper Position"=0, "z Stepper Position"=0} -> [w210]
    shift-right: [w205] -> _
    shift-left: T11 {"Yaw"=0.0, "Compass"=0.0} -> [w207]
    shift-right: [w202] -> _
    shift-left: T10 {"Time up flag"=FALSE, "SET TIME TO CHECK"=0.0} -> [w204]
    shift-right: [w200] -> _
    shift-left: T9 {"yStepper desired"=0} -> [w201]
    shift-right: [w196] -> _
    shift-left: T8 {"Left IR Sensor"=0.0, "Arm IR Sensor"=0.0, "Bottom IR Sensor"=0.0} -> [w198]
    stop <- w229 stop-if-true
    # ">>> yStepper command>>>"
    # ">>True Stop Next State >>"
    # ">>Error  >>"
    # ">>Timeout>>"
    # ">>Action states Queue Reference >>"
    # ">>State Logic Queue Reference >>"
    # "TOP LEVEL BASELINE (MAIN PROCESSING LOOP)"
    n58 = Dequeue Element(queue=w242, timeout in ms (-1)=0, error in (no error)=w240) -> (queue out=w234:refnum<queue>, element=w241:string, error out=w235:errorcluster)  [unwired: 1 out]
    "Action State" <- w241
    n59 = Wait (ms)(milliseconds to wait=u32 20) -> ()  [unwired: 1 out]
    n60 = case shown="\"R-ACW\"" w241 {
      tunnel: [_ _ _ _ _ _ _ _ _ _ _ _ _ _ _ _ _ _ 0 w1376 _ _ _ _ _ _ _ _ _ _ _ _ _ _ _ _ _ _ _ _ _ _] -> w237
      tunnel: w234 -> [_ _ _ _ _ _ _ _ _ _ _ _ _ _ _ _ _ _ _ _ _ _ _ _ _ _ _ _ _ _ _ _ _ _ _ _ _ _ _ _ _ _]
      tunnel: w233 -> [w1147 w1156 w1168 w1179 w1196 w1207 w1218 w1230 w1242 w1253 w1260 w1275 w1289 w1301 w1309 w1321 w1346 w1356 w1367 w1377 w1386 w1396 w1426 w1437 w1445 w1454 w1467 w1480 w1490 w1499 w1516 w1525 w1536 w1546 w1556 w1566 w1573 w1585 w1601 w1607 w1619 w1630]
      tunnel: [w1147 w1156 w1168 w1179 w1196 w1207 w1218 w1230 w1242 w1253 w1260 w1275 w1290 w1301 w1309 w1321 w1347 w1356 w1367 w1377 w1386 w1396 w1425 w1437 w1445 w1454 w1467 w1480 w1490 w1499 w1516 w1525 w1536 w1546 w1556 w1566 w1573 w1585 w1601 w1607 w1619 w1630] -> w232
      tunnel: [TRUE TRUE _ _ _ _ _ _ _ _ _ _ _ _ _ _ _ _ _ _ _ _ _ _ _ _ _ _ _ _ _ _ _ _ _ _ _ _ _ _ _ _] -> w229
      tunnel: w227 -> [w1145 w1154 w1167 w1178 w1195 w1206 w1217 w1229 w1241 w1252 w1259 w1274 w1288 w1300 w1307 w1320 w1345 w1355 w1364 w1374 w1385 w1395 w1424 w1436 w1444 w1453 w1466 w1479 w1489 w1498 w1515 w1524 w1535 w1545 w1555 w1565 w1572 w1584 w1600 w1606 w1618 w1629]
      tunnel: [_ _ _ _ _ _ _ _ _ _ _ _ _ _ _ _ _ _ _ TRUE _ _ _ _ _ _ _ _ _ _ _ _ _ _ _ _ _ _ _ _ _ _] -> w226
      tunnel: [w1145 w1154 w1167 w1178 w1195 w1206 w1217 w1229 w1241 w1252 w1259 w1274 w1288 w1300 w1307 w1320 w1345 w1355 w1364 w1374 w1385 w1395 w1424 w1436 w1444 w1453 w1466 w1479 w1489 w1498 w1515 w1524 w1535 w1545 w1555 w1565 w1572 w1584 w1600 w1606 w1618 w1629] -> w225
      tunnel: w222 -> [w1144 w1153 w1166 w1181 w1194 w1205 w1216 w1228 w1240 w1251 w1261 w1273 w1287 w1302 w1311 w1322 w1344 w1357 w1363 w1373 w1387 w1397 w1414 w1435 w1447 w1455 w1468 w1481 w1491 w1500 w1517 w1527 w1538 w1548 w1558 w1568 w1575 w1587 w1603 w1609 w1621 w1632]
      tunnel: [w1144 w1153 w1166 w1181 w1194 w1205 w1216 w1228 w1240 w1251 w1261 w1272 w1287 w1302 w1311 w1322 w1343 w1357 w1363 w1373 w1387 w1397 w1413 w1435 w1447 w1455 w1468 w1481 w1491 w1500 w1517 w1527 w1538 w1548 w1558 w1568 w1575 w1587 w1603 w1609 w1621 w1632] -> w221
      tunnel: w215 -> [w1139 _ _ _ _ _ _ _ _ _ _ _ _ _ _ _ _ _ _ _ _ _ _ _ _ _ _ _ _ _ w1511 _ _ _ _ _ _ _ _ _ _ _]
      tunnel: w214 -> [_ _ _ _ _ _ _ _ _ _ _ _ _ _ _ _ _ _ _ _ _ _ _ _ _ _ _ _ w1483 _ w1513 w1523 _ _ _ _ _ _ _ _ _ _]
      tunnel: w213 -> [w1143 w1152 w1165 w1180 w1193 w1204 w1215 w1227 w1239 w1249 w1258 w1271 w1286 w1295 w1310 w1319 w1335 w1354 w1362 w1372 w1384 w1394 w1419 w1433 w1446 w1452 w1465 w1478 w1485 w1497 w1508 w1526 w1537 w1547 w1557 w1567 w1574 w1586 w1602 w1608 w1620 w1631]
      tunnel: [w1143 w1152 w1165 w1180 w1193 w1204 w1215 w1227 w1239 w1249 w1258 w1271 w1286 w1295 w1310 w1319 w1334 w1354 w1362 w1372 w1384 w1394 w1418 w1433 w1446 w1452 w1465 w1478 w1485 w1497 w1507 w1526 w1537 w1547 w1557 w1567 w1574 w1586 w1602 w1608 w1620 w1631] -> w212
      tunnel: w210 -> [w1142 w1151 w1164 w1182 w1192 w1203 w1214 w1226 w1238 w1248 w1257 w1270 w1285 w1303 w1312 w1318 w1340 w1353 w1361 w1371 w1383 w1393 w1409 w1432 w1443 w1451 w1464 w1477 w1488 w1496 w1518 w1528 w1534 w1544 w1554 w1564 w1576 w1588 w1599 w1610 w1622 w1633]
      tunnel: [w1142 w1151 w1164 w1182 w1192 w1203 w1214 w1226 w1238 w1248 w1257 w1270 w1285 w1303 w1312 w1318 w1339 w1353 w1361 w1371 w1383 w1393 w1408 w1432 w1443 w1451 w1464 w1477 w1488 w1496 w1518 w1528 w1534 w1544 w1554 w1564 w1576 w1588 w1598 w1610 w1622 w1633] -> w209
      tunnel: w207 -> [w1141 w1150 w1162 w1183 w1190 w1201 w1213 w1224 w1236 w1247 w1256 w1269 w1278 w1298 w1313 w1317 w1330 w1352 w1360 w1370 w1382 w1392 w1405 w1431 w1440 w1450 w1463 w1476 w1487 w1495 w1519 w1529 w1533 w1541 w1551 w1561 w1577 w1589 w1593 w1611 w1623 w1634]
      tunnel: [w1141 w1150 w1162 w1183 w1190 w1201 w1213 w1224 w1236 w1247 w1256 w1269 w1278 w1297 w1313 w1317 w1329 w1352 w1360 w1370 w1382 w1392 w1404 w1431 w1440 w1450 w1463 w1476 w1487 w1495 w1519 w1529 w1533 w1541 w1551 w1561 w1577 w1589 w1593 w1611 w1623 w1634] -> w206
      tunnel: w204 -> [w1138 w1149 w1163 w1184 w1191 w1202 w1212 w1225 w1237 w1246 w1255 w1268 w1277 w1294 w1314 w1316 w1326 w1349 w1359 w1369 w1381 w1391 w1402 w1429 w1439 w1449 w1462 w1475 w1486 w1494 w1520 w1530 w1532 w1540 w1550 w1560 w1578 w1590 w1592 w1605 w1617 w1628]
      tunnel: [w1138 w1149 w1163 w1184 w1191 w1202 w1212 w1225 w1237 w1246 w1255 w1268 w1277 w1294 w1314 w1316 w1326 w1349 w1359 w1369 w1381 w1391 w1401 w1429 w1439 w1449 w1462 w1475 w1486 w1494 w1520 w1530 w1532 w1540 w1550 w1560 w1578 w1590 w1592 w1605 w1615 w1627] -> w203
      tunnel: w201 -> [_ _ _ _ _ _ _ _ _ _ _ _ _ _ _ _ _ _ _ _ _ _ _ _ _ _ _ _ _ _ _ _ _ _ _ _ _ w1581 _ _ _ _]
      tunnel: [w1137 w1148 w1157 w1174 w1185 w1197 w1208 w1219 w1231 w1243 w1254 w1262 w1276 w1291 w1305 w1315 w1323 w1348 w1358 w1368 w1380 w1388 w1398 w1428 w1438 w1448 w1456 w1469 w1482 w1492 w1501 w1521 w1531 w1539 w1549 w1559 w1569 w1579 w1591 w1604 w1612 w1624] -> w197
      tunnel: w198 -> [w1137 w1148 w1157 w1174 w1185 w1197 w1208 w1219 w1231 w1243 w1254 w1262 w1276 w1291 w1306 w1315 w1323 w1348 w1358 w1368 w1380 w1388 w1398 w1428 w1438 w1448 w1456 w1469 w1482 w1492 w1501 w1521 w1531 w1539 w1549 w1559 w1569 w1579 w1591 w1604 w1612 w1624]
      frame "Exit" {
        # ">>State Logic  >>"
        # ">>> Time cluster >>>"
        # ">>> Yaw >>>"
        # ">>> Stepper position >>>"
        # ">>> Encoders >>>"
        # ">>> Object detection >>>"
        # ">>> Ultrasonic Sensors Detect >>>"
        n61 = call "Imaq Dispose"("All Images? (No)"=TRUE, "Image"=w1139) -> ()  [unwired: 4 in, 1 out]
      }
      frame "----Movement States----" {
        # ">>State Logic  >>"
        # ">>> Time cluster >>>"
        # ">>> Yaw >>>"
        # ">>> Stepper position >>>"
        # ">>> Encoders >>>"
        # ">>> Object detection >>>"
        # ">>> Ultrasonic Sensors Detect >>>"
      }
      frame "FORWARD" {
        # ">>State Logic  >>"
        # ">>> Time cluster >>>"
        # ">>> Yaw >>>"
        # ">>> Stepper position >>>"
        # ">>> Encoders >>>"
        # ">>> Object detection >>>"
        # ">>> Ultrasonic Sensors Detect >>>"
        n62 = Unbundle By Name(w1162) -> ("Yaw"=w1158:dbl)
        n63 = call "MOTOR CONTROL WITH PID AE.vi"("Yaw"=w1158, "Speed"=50.0, "Direction"=MOTOR_CONTROL_WITH_PID_AE_DIRECTION_TYPE_DEF."y-axis movement", "AE Mode"=MOTOR_CONTROL_WITH_PID_AE_DATA_MODE_TYPE_DEF."Write to AE") -> ()  [unwired: 1 out]
      }
      frame "FORWARD - IR ASSIST" {
        # ">>State Logic  >>"
        # ">>> Time cluster >>>"
        # ">>> Yaw >>>"
        # ">>> Stepper position >>>"
        # ">>> Encoders >>>"
        # ">>> Object detection >>>"
        # ">>> Ultrasonic Sensors Detect >>>"
        n64 = Unbundle By Name(w1174) -> ("Left IR Sensor"=w1173:dbl)
        n65 = Subtract(x=w1173, y=20.0) -> (x-y=w1171:dbl)
        n66 = Multiply(x=w1171, y=0.2) -> (x*y=w1169:dbl)
        n67 = call "MOTOR CONTROL WITH PID AE.vi"("Yaw"=w1169, "Speed"=30.0, "Direction"=MOTOR_CONTROL_WITH_PID_AE_DIRECTION_TYPE_DEF."y-axis movement", "AE Mode"=MOTOR_CONTROL_WITH_PID_AE_DATA_MODE_TYPE_DEF."Write to AE") -> ()  [unwired: 1 out]
      }
      frame "LEFT" {
        # ">>State Logic  >>"
        # ">>> Time cluster >>>"
        # ">>> Yaw >>>"
        # ">>> Stepper position >>>"
        # ">>> Encoders >>>"
        # ">>> Object detection >>>"
        # ">>> Ultrasonic Sensors Detect >>>"
        n68 = Unbundle By Name(w1190) -> ("Yaw"=w1187:dbl)
        n69 = call "MOTOR CONTROL WITH PID AE.vi"("Yaw"=w1187, "Speed"=-25.0, "Direction"=MOTOR_CONTROL_WITH_PID_AE_DIRECTION_TYPE_DEF."x-axis movement", "AE Mode"=MOTOR_CONTROL_WITH_PID_AE_DATA_MODE_TYPE_DEF."Write to AE") -> ()  [unwired: 1 out]
      }
      frame "R-ACW" {
        # ">>> IR Sensors >>>"
        # ">>> Time cluster >>>"
        # ">>> Yaw >>>"
        # ">>> Stepper position >>>"
        # ">>> Encoders >>>"
        # ">>> Object detection >>>"
        # ">>> Ultrasonic Sensors Detect >>>"
        n70 = call "MOTOR CONTROL WITH PID AE.vi"("Speed"=80.0, "Direction"=MOTOR_CONTROL_WITH_PID_AE_DIRECTION_TYPE_DEF."rotation", "AE Mode"=MOTOR_CONTROL_WITH_PID_AE_DATA_MODE_TYPE_DEF."Write to AE") -> ()  [unwired: 1 in, 1 out]
      }
      frame "R-CW" {
        (unwired) -0.2 ("Speed")
        # ">>> Time cluster >>>"
        # ">>> Yaw >>>"
        # ">>> Stepper position >>>"
        # ">>> Encoders >>>"
        # ">>> Object detection >>>"
        # ">>> Ultrasonic Sensors Detect >>>"
        n71 = call "MOTOR CONTROL WITH PID AE.vi"("Speed"=60.0, "Direction"=MOTOR_CONTROL_WITH_PID_AE_DIRECTION_TYPE_DEF."rotation", "AE Mode"=MOTOR_CONTROL_WITH_PID_AE_DATA_MODE_TYPE_DEF."Write to AE") -> ()  [unwired: 1 in, 1 out]
      }
      frame "RIGHT" {
        # ">>> Time cluster >>>"
        # ">>> Yaw >>>"
        # ">>> Stepper position >>>"
        # ">>> Encoders >>>"
        # ">>> Object detection >>>"
        # ">>> Ultrasonic Sensors Detect >>>"
        n72 = Unbundle By Name(w1224) -> ("Yaw"=w1220:dbl)
        n73 = call "MOTOR CONTROL WITH PID AE.vi"("Yaw"=w1220, "Speed"=50.0, "Direction"=MOTOR_CONTROL_WITH_PID_AE_DIRECTION_TYPE_DEF."x-axis movement", "AE Mode"=MOTOR_CONTROL_WITH_PID_AE_DATA_MODE_TYPE_DEF."Write to AE") -> ()  [unwired: 1 out]
      }
      frame "REVERSE" {
        # ">>> Time cluster >>>"
        # ">>> Yaw >>>"
        # ">>> Stepper position >>>"
        # ">>> Encoders >>>"
        # ">>> Object detection >>>"
        # ">>> Ultrasonic Sensors Detect >>>"
        n74 = Unbundle By Name(w1236) -> ("Yaw"=w1232:dbl)
        n75 = call "MOTOR CONTROL WITH PID AE.vi"("Yaw"=w1232, "Speed"=-50.0, "Direction"=MOTOR_CONTROL_WITH_PID_AE_DIRECTION_TYPE_DEF."y-axis movement", "AE Mode"=MOTOR_CONTROL_WITH_PID_AE_DATA_MODE_TYPE_DEF."Write to AE") -> ()  [unwired: 1 out]
      }
      frame "STOP" {
        n76 = Wait (ms)(milliseconds to wait=u32 100) -> ()  [unwired: 1 out]
        n77 = call "MOTOR CONTROL WITH PID AE.vi"("Direction"=MOTOR_CONTROL_WITH_PID_AE_DIRECTION_TYPE_DEF."stop", "AE Mode"=MOTOR_CONTROL_WITH_PID_AE_DATA_MODE_TYPE_DEF."Write to AE") -> ()  [unwired: 2 in, 1 out]
      }
      frame "----SENSOR READING---- " {
      }
      frame "READ ENCODERS" {
        # ">>> Time cluster >>>"
        # ">>> Yaw >>>"
        # ">>> Stepper position >>>"
        # ">>> Object detection >>>"
        # ">>> Current encoder distance >>>"
        # ">>> Ultrasonic Sensors Detect >>>"
        n78 = call "MOTOR CONTROL WITH PID AE.vi"("AE Mode"=MOTOR_CONTROL_WITH_PID_AE_DATA_MODE_TYPE_DEF."Read from AE") -> ("Speed & distance"=w1266:T1)  [unwired: 3 in]
        n79 = Unbundle By Name(w1266) -> ("xDistance"=w1265:dbl, "yDistance"=w1264:dbl, "wDistance"=w1263:dbl)
        n80 = Bundle By Name(cluster=w1273, "xDistance"=w1265, "yDistance"=w1264, "wDistance"=w1263) -> (w1272:T16)
      }
      frame "READ ULTRASONIC" {
        (unwired) navX_type_def."Read Values" ("Mode")
        (unwired) MOTOR_CONTROL_NO_PID_Type_Def."Latch" ("Direction")
        # ">>State Logic  >>"
        # ">>> Time cluster >>>"
        # ">>> Ultrasonic Sensors Detect >>>"
        # ">>> Object detection >>>"
        # ">>> Encoders >>>"
        # ">>> Stepper position >>>"
        # ">>> Yaw >>>"
        n81 = call "Arduino Interfacing VI.vi"("AE Mode"=Arduino_Interfacing."Read From Arduino") -> ("Arduino Data"=w1283:T4)  [unwired: 3 in, 1 out]
        n82 = Unbundle By Name(w1283) -> ("PING A"=w1282:u8, "PING B"=w1281:u8, "PING C"=w1280:u8, "PING D"=w1279:u8)
        n83 = Bundle By Name(cluster=w1289, "PING_A"=w1282, "PING_B"=w1281, "PING_C"=w1280, "PING_D"=w1279) -> (w1290:T15)
      }
      frame "READ NAVX" {
        # ">>> Time cluster >>>"
        # ">>> Yaw >>>"
        # ">>> Ultrasonic Sensors Detect >>>"
        # ">>> Object detection >>>"
        # ">>> Encoders >>>"
        # ">>> Stepper position >>>"
        n84 = call "navX reading VI.vi"("Mode"=navX_type_def."Read Values") -> ("NavX Readings"=w1293:T3)  [unwired: 2 in, 3 out]
        n85 = Unbundle By Name(w1293) -> ("Heading"=w1292:dbl)
        n86 = Unbundle By Name(w1293) -> ("Yaw"=w1296:dbl)
        n87 = Bundle By Name(cluster=w1298, "Yaw"=w1296, "Compass"=w1292) -> (w1297:T11)
      }
      frame "READ IR" {
        w1308 = T33 [enum."A/AI0"] items=["Not Connected", "AudioIn/Left", "AudioIn/Right", "C/AI0", "C/AI1", "A/AI0", "A/AI1", "A/AI2", "A/AI3", "A/AI4", "A/AI5", "A/AI6", "A/AI7", "B/AI0", "B/AI1", "B/AI2", "B/AI3", "B/AI4", "B/AI5", "B/AI6", "B/AI7", "AI/AI0", "AI/AI1", "AI/AI2", "AI/AI3", "A/AI0 (DIFF)", "A/AI1 (DIFF)", "A/AI2 (DIFF)", "A/AI3 (DIFF)", "B/AI0 (DIFF)", "B/AI1 (DIFF)", "B/AI2 (DIFF)", "B/AI3 (DIFF)"] ("AI Channel")
        # ">>State Logic  >>"
        # ">>> Time cluster >>>"
        # ">>> Ultrasonic Sensors Detect >>>"
        # ">>> Object detection >>>"
        # ">>> Encoders >>>"
        # ">>> Stepper position >>>"
        # ">>> Yaw >>>"
        n88 = call <vilib>:"Sharp IR.vi"("AI Channel"=w1308) -> ("Sharp IR Distance"=w1304:dbl)  [unwired: 8 in, 2 out]
        n89 = Bundle By Name(cluster=w1306, "Left IR Sensor"=w1304) -> (w1305:T8)
      }
      frame "----SYSTEM MODES----" {
        (unwired) I2C_MASTER_Type_Def."Last State" ("Arduino Mode")
        # ">>> Object detection >>>"
        # ">>> Yaw >>>"
        # ">>> Ultrasonic Sensors Detect >>>"
        # ">>> Encoders >>>"
        # ">>> Stepper position >>>"
      }
      frame "INIT" {
        w1341 = u8 0
        w1342 = 0.0
        # ">>> Time cluster >>>"
        # ">>> Object detection >>>"
        # ">>> Yaw >>>"
        # ">>> Ultrasonic Sensors Detect >>>"
        # ">>> Encoders >>>"
        # ">>> Stepper position >>>"
        # ">>State Logic  >>"
        n90 = call "Arduino Interfacing VI.vi"("AE Mode"=Arduino_Interfacing."Initialize") -> ()  [unwired: 3 in, 2 out]
        n91 = call "FGV Bool.vi"("Init/Read/Write State"=States_for_Action_Engine."Initialize") -> ()  [unwired: 2 in, 2 out]
        n92 = call "Elasped Timer.vi"("Action"=Elapsed_timer_control."Initialize") -> ()  [unwired: 7 in, 4 out]
        n93 = call "MOTOR CONTROL WITH PID AE.vi"("AE Mode"=MOTOR_CONTROL_WITH_PID_AE_DATA_MODE_TYPE_DEF."Init AE") -> ()  [unwired: 3 in, 1 out]
        n94 = Bundle By Name(cluster=w1335, "Recognized Object"=FALSE, "Object X coordinate"=0.0, "Object Y coordinate"=0.0) -> (w1334:T14)
        n95 = Bundle By Name(cluster=w1340, "y Stepper Position"=u8 0, "z Stepper Position"=u8 0) -> (w1339:T12)
        n96 = Bundle By Name(cluster=w1344, "xDistance"=w1342, "yDistance"=w1342, "wDistance"=w1342) -> (w1343:T16)
        n97 = Bundle By Name(cluster=w1346, "PING_A"=w1341, "PING_B"=w1341, "PING_C"=w1341, "PING_D"=w1341) -> (w1347:T15)
        n98 = Bundle By Name(cluster=w1330, "Yaw"=0.0) -> (w1329:T11)
      }
      frame "ARDUINO - ULTRASONIC" {
        # ">>> Object detection >>>"
        # ">>> Yaw >>>"
        # ">>> Ultrasonic Sensors Detect >>>"
        # ">>> Encoders >>>"
        # ">>> Stepper position >>>"
        # ">>State Logic  >>"
        n99 = call "Arduino Interfacing VI.vi"("Data to Write"=I2C_MASTER_WRITE_NEW_Type_Def."Ultrasonic sensors", "AE Mode"=Arduino_Interfacing."Write to Arduino") -> ()  [unwired: 2 in, 2 out]
      }
      frame "NAVX CALIBRATE" {
        # ">>> Object detection >>>"
        # ">>> Yaw >>>"
        # ">>> Ultrasonic Sensors Detect >>>"
        # ">>> Encoders >>>"
        # ">>> Stepper position >>>"
        # ">>State Logic  >>"
        # "Adds a 15 second delay to the startup process \nfor the NavX to calibrate"
        n100 = Wait (ms)(milliseconds to wait=u32 5000) -> ()  [unwired: 1 out]
      }
      frame "NO ACTION", Default {
        (unwired) u8 0 ("y Stepper value")
        (unwired) TRUE ("Latch")
        (unwired) navX_type_def."Read Values" ("Mode")
        (unwired) MOTOR_CONTROL_NO_PID_Type_Def."Latch" ("Direction")
        # ">>> Object detection >>>"
        # ">>> Yaw >>>"
        # ">>> Ultrasonic Sensors Detect >>>"
        # ">>> Encoders >>>"
        # ">>> Stepper position >>>"
        # ">>State Logic  >>"
        n101 = case shown="4" w1374 {
          tunnel: [0 100] -> w1376
          frame 1, Default {
          }
          frame 4 {
          }
        }
      }
      frame "----RESET CASES----" {
        (unwired) I2C_MASTER_Type_Def."Last State" ("Arduino Mode")
        # ">>> Object detection >>>"
        # ">>> Yaw >>>"
        # ">>> Ultrasonic Sensors Detect >>>"
        # ">>> Encoders >>>"
        # ">>> Stepper position >>>"
        # ">>State Logic  >>"
      }
      frame "RESET ENCODERS" {
        # ">>> Object detection >>>"
        # ">>> Yaw >>>"
        # ">>> Ultrasonic Sensors Detect >>>"
        # ">>> Encoders >>>"
        # ">>> Stepper position >>>"
        # ">>State Logic  >>"
        n102 = call "MOTOR CONTROL WITH PID AE.vi"("Direction"=MOTOR_CONTROL_WITH_PID_AE_DIRECTION_TYPE_DEF."reset encoders", "AE Mode"=MOTOR_CONTROL_WITH_PID_AE_DATA_MODE_TYPE_DEF."Write to AE") -> ()  [unwired: 2 in, 1 out]
      }
      frame "RESET FLAGS" {
        (unwired) I2C_MASTER_Type_Def."Last State" ("Arduino Mode")
        # "Resets any software variables\nand/or non-critical states"
        n103 = Wait (ms)(milliseconds to wait=u32 20) -> ()  [unwired: 1 out]
        n104 = Bundle By Name(cluster=w1402, "Time up flag"=FALSE, "SET TIME TO CHECK"=0.0) -> (w1401:T10)
        n105 = Bundle By Name(cluster=w1419, "Recognized Object"=FALSE, "Object X coordinate"=0.0, "Object Y coordinate"=0.0) -> (w1418:T14)
        n106 = Bundle By Name(cluster=w1409, "y Stepper Position"=u8 0, "z Stepper Position"=u8 0) -> (w1408:T12)
        n107 = Bundle By Name(cluster=w1414, "xDistance"=0.0, "yDistance"=0.0, "wDistance"=0.0) -> (w1413:T16)
        n108 = Bundle By Name(cluster=w1426, "PING_A"=u8 0, "PING_B"=u8 0, "PING_C"=u8 0, "PING_D"=u8 0) -> (w1425:T15)
        n109 = Bundle By Name(cluster=w1405, "Yaw"=0.0) -> (w1404:T11)
      }
      frame "RESET YAW" {
        n110 = Wait (ms)(milliseconds to wait=u32 100) -> ()  [unwired: 1 out]
        n111 = call "navX reading VI.vi"("Mode"=navX_type_def."Zero Yaw") -> ()  [unwired: 2 in, 4 out]
      }
      frame "RESET ARM" {
        n112 = call "Arduino Interfacing VI.vi"("Data to Write"=I2C_MASTER_WRITE_NEW_Type_Def."Soft Reset", "AE Mode"=Arduino_Interfacing."Write to Arduino") -> ()  [unwired: 2 in, 2 out]
      }
      frame "--------CAM STATES-------" {
      }
      frame "OPEN LOG CAM" {
        n113 = call "Webcam AE.vi"("Session In"=T30 "cam0", "Camera states"=Webcam_AE."Initialize Camera") -> ("error out"=w1459:errorcluster, "Session Out"=w1458:T30)  [unwired: 1 in, 1 out]
        n114 = call "Webcam AE.vi"("error in (no error)"=w1459, "Session In"=w1458, "Camera states"=Webcam_AE."Open Camera") -> ()  [unwired: 3 out]
      }
      frame "OPEN LIFE CAM" {
        n115 = call "Webcam AE.vi"("Session In"=T30 "cam1", "Camera states"=Webcam_AE."Initialize Camera") -> ("error out"=w1472:errorcluster, "Session Out"=w1471:T30)  [unwired: 1 in, 1 out]
        n116 = call "Webcam AE.vi"("error in (no error)"=w1472, "Session In"=w1471, "Camera states"=Webcam_AE."Open Camera") -> ()  [unwired: 3 out]
      }
      frame "CAM ACQ" {
        # ">>State Logic  >>"
        # ">>> Time cluster >>>"
        # ">>> Yaw >>>"
        # ">>> Stepper position >>>"
        # ">>> Encoders >>>"
        # ">>> Object detection >>>"
        # ">>> Ultrasonic Sensors Detect >>>"
        n117 = call "Webcam AE.vi"("error in (no error)"=w1483, "Camera states"=Webcam_AE."Continuous Acquisition") -> ()  [unwired: 1 in, 3 out]
      }
      frame "CAM CLOSE" {
        # ">>State Logic  >>"
        # ">>> Time cluster >>>"
        # ">>> Yaw >>>"
        # ">>> Stepper position >>>"
        # ">>> Encoders >>>"
        # ">>> Object detection >>>"
        # ">>> Ultrasonic Sensors Detect >>>"
        n118 = call "Webcam AE.vi"("Camera states"=Webcam_AE."Close Camera") -> ()  [unwired: 2 in, 3 out]
      }
      frame "PROCESS IMAGE" {
        # ">>State Logic  >>"
        # ">>> Time cluster >>>"
        # ">>> Yaw >>>"
        # ">>> Stepper position >>>"
        # ">>> Encoders >>>"
        # ">>> Object detection >>>"
        # ">>> Ultrasonic Sensors Detect >>>"
        n119 = call "Webcam AE.vi"("error in (no error)"=w1513, "Camera states"=Webcam_AE."Retrieve Image") -> ("error out"=w1509:errorcluster, "Image Out"=w1512:T23)  [unwired: 1 in, 1 out]
        n120 = call "Object Detection SubVI.vi"("Error In"=w1509, "Mode"="Object recognition mode", "Image Dest"=w1511, "Image in"=w1512) -> ("Object Center Coordinates"=w1506:cluster{"x":sgl, "y":sgl}, "Object detection cluster"=w1502:T2)  [unwired: 2 out]
        "Object detection cluster" <- w1502
        "Object Center Coordinates" <- w1506
        n121 = Unbundle By Name(w1502) -> ("Object detected?"=w1503:bool)
        n122 = Unbundle By Name(w1506) -> ("x"=w1505:sgl, "y"=w1504:sgl)
        n123 = Bundle By Name(cluster=w1508, "Recognized Object"=w1503, "Object X coordinate"=w1505, "Object Y coordinate"=w1504) -> (w1507:T14)
      }
      frame "DISPOSE BUFFERS" {
        # ">>State Logic  >>"
        # ">>> Time cluster >>>"
        # ">>> Yaw >>>"
        # ">>> Stepper position >>>"
        # ">>> Encoders >>>"
        # ">>> Object detection >>>"
        # ">>> Ultrasonic Sensors Detect >>>"
        n124 = call "Webcam AE.vi"("error in (no error)"=w1523, "Camera states"=Webcam_AE."Dispose Image Buffers") -> ()  [unwired: 1 in, 3 out]
      }
      frame "-----ARM ACTIONS-----" {
      }
      frame "CLOSE CLAW" {
        n125 = call "Arduino Interfacing VI.vi"("Data to Write"=I2C_MASTER_WRITE_NEW_Type_Def."Close Claw", "AE Mode"=Arduino_Interfacing."Write to Arduino") -> ()  [unwired: 2 in, 2 out]
      }
      frame "OPEN CLAW" {
        n126 = call "Arduino Interfacing VI.vi"("Data to Write"=I2C_MASTER_WRITE_NEW_Type_Def."Open Claw", "AE Mode"=Arduino_Interfacing."Write to Arduino") -> ()  [unwired: 2 in, 2 out]
      }
      frame "Z STEPPER CAM HEIGHT" {
        n127 = call "Arduino Interfacing VI.vi"("Data to Write"=I2C_MASTER_WRITE_NEW_Type_Def."zStepper 8k", "AE Mode"=Arduino_Interfacing."Write to Arduino") -> ()  [unwired: 2 in, 2 out]
      }
      frame "Z STEPPER GRAB HEIGHT" {
        # ">>State Logic  >>"
        # ">>> Time cluster >>>"
        # ">>> Yaw >>>"
        # ">>> Stepper position >>>"
        # ">>> Encoders >>>"
        # ">>> Object detection >>>"
        # ">>> Ultrasonic Sensors Detect >>>"
        n128 = call "Arduino Interfacing VI.vi"("Data to Write"=I2C_MASTER_WRITE_NEW_Type_Def."zStepper 100", "AE Mode"=Arduino_Interfacing."Write to Arduino") -> ()  [unwired: 2 in, 2 out]
      }
      frame "Y STEPPER CONTROL" {
        # ">>State Logic  >>"
        # ">>> yStepper command>>>"
        # ">>> Time cluster >>>"
        # ">>> Yaw >>>"
        # ">>> Stepper position >>>"
        # ">>> Encoders >>>"
        # ">>> Object detection >>>"
        # ">>> Ultrasonic Sensors Detect >>>"
        n129 = Unbundle By Name(w1581) -> ("yStepper desired"=w1580:u8)
        n130 = call "Arduino Interfacing VI.vi"("y Stepper value"=w1580, "Data to Write"=I2C_MASTER_WRITE_NEW_Type_Def."yStepper control", "AE Mode"=Arduino_Interfacing."Write to Arduino") -> ()  [unwired: 1 in, 2 out]
      }
      frame "READ STEPPER VALUES" {
        # ">>State Logic  >>"
        # ">>> Time cluster >>>"
        # ">>> Yaw >>>"
        # ">>> Stepper position >>>"
        # ">>> Encoders >>>"
        # ">>> Object detection >>>"
        # ">>> Ultrasonic Sensors Detect >>>"
        n131 = call "Arduino Interfacing VI.vi"("AE Mode"=Arduino_Interfacing."Read From Arduino") -> ("Arduino Data"=w1596:T4)  [unwired: 3 in, 1 out]
        n132 = Unbundle By Name(w1596) -> ("y Stepper Position"=w1595:u8, "z Stepper Position"=w1594:u8)
        n133 = Bundle By Name(cluster=w1599, "y Stepper Position"=w1595, "z Stepper Position"=w1594) -> (w1598:T12)
      }
      frame " -----TIMING-----" {
        # ">>State Logic  >>"
        # ">>> Time cluster >>>"
        # ">>> Yaw >>>"
        # ">>> Stepper position >>>"
        # ">>> Encoders >>>"
        # ">>> Object detection >>>"
        # ">>> Ultrasonic Sensors Detect >>>"
      }
      frame "SET TIMER" {
        # ">>State Logic  >>"
        # ">>> Time cluster >>>"
        # ">>> Yaw >>>"
        # ">>> Stepper position >>>"
        # ">>> Encoders >>>"
        # ">>> Object detection >>>"
        # ">>> Ultrasonic Sensors Detect >>>"
        n134 = call "Elasped Timer.vi"("Time Setting"=5.0, "Action"=Elapsed_timer_control."Initialize") -> ()  [unwired: 6 in, 4 out]
        n135 = Bundle By Name(cluster=w1617, "Time up flag"=FALSE) -> (w1615:T10)
      }
      frame "START TIMER" {
        # ">>State Logic  >>"
        # ">>> Time cluster >>>"
        # ">>> Yaw >>>"
        # ">>> Stepper position >>>"
        # ">>> Encoders >>>"
        # ">>> Object detection >>>"
        # ">>> Ultrasonic Sensors Detect >>>"
        n136 = call "Elasped Timer.vi"("Action"=Elapsed_timer_control."Start") -> ("Time Out?!"=w1625:bool)  [unwired: 7 in, 3 out]
        n137 = Bundle By Name(cluster=w1628, "Time up flag"=w1625) -> (w1627:T10)
      }
    }
    "State Logic" <- w225
    n138 = local read "TASK ENABLE"() -> (w219:bool)
    n139 = Not(x=w219) -> (.not. x?=w218:bool)
    n140 = case shown="True" w226 {
      tunnel: w230 -> [w254 w287]
      tunnel: w234 -> [w250 w289]
      tunnel: [w254 w287] -> w239
      tunnel: [w250 w290] -> w238
      tunnel: w235 -> [_ w285]
      tunnel: w237 -> [_ w286]
      tunnel: w232 -> [w253 w292]
      tunnel: [w253 w292] -> w231
      tunnel: "STOP TASK" -> [_ w275]
      tunnel: w225 -> [w252 w291]
      tunnel: [w252 w288] -> w224
      tunnel: w221 -> [w251 w281]
      tunnel: [w251 w281] -> w220
      tunnel: w218 -> [_ w276]
      tunnel: [w249 w273] -> w217
      tunnel: w216 -> [w249 w272]
      tunnel: w212 -> [w248 w269]
      tunnel: [w248 w269] -> w211
      tunnel: w209 -> [w247 w265]
      tunnel: [w247 w265] -> w208
      tunnel: w206 -> [w246 w263]
      tunnel: [w246 w263] -> w205
      tunnel: w203 -> [w245 w261]
      tunnel: [w245 w261] -> w202
      tunnel: w201 -> [w244 w260]
      tunnel: [w244 w259] -> w200
      tunnel: [_ w257] -> w199
      tunnel: w197 -> [w243 w255]
      tunnel: [w243 w255] -> w196
      frame False {
        # ">>> IR Sensors >>>"
        # ">>> IR Sensors >>>"
        # ">>> yStepper command>>>"
        # ">>> Time cluster >>>"
        # ">>> Yaw >>>"
        # ">>> Stepper position >>>"
        # ">>> Encoders >>>"
        # ">>> Object detection >>>"
        # ">>> Ultrasonic Sensors Detect >>>"
        # ">>> Time cluster >>>"
        # ">>> Yaw >>>"
        # ">>> Stepper position >>>"
        # ">>> Encoders >>>"
        # ">>> Object detection >>>"
        # ">>> Ultrasonic Sensors Detect >>>"
      }
      frame True {
        # ">>State Logic Queue Reference >>"
        # ">>Timeout>>"
        # ">>> yStepper command>>>"
        # ">>> Time cluster >>>"
        # ">>> Object detection >>>"
        # ">>> Yaw >>>"
        # ">>> Ultrasonic Sensors Detect >>>"
        # ">>> Encoders >>>"
        # ">>> Stepper position >>>"
        # ">>State Logic  >>"
        # ">>True Stop Next State >>"
        # ">>Action Queue>>"
        # ">> Manual override >>"
        # ">>> Time cluster >>>"
        # ">>> Yaw >>>"
        # ">>> Stepper position >>>"
        # ">>> Encoders >>>"
        # ">>> Object detection >>>"
        # ">>> Ultrasonic Sensors Detect >>>"
        # ">>Action Queue>>"
        # ">>State Logic Queue Reference >>"
        n141 = Or(x=w275, y=w276) -> (x .or. y?=w274:bool)
        n142 = Unbundle By Name(w255) -> ("Left IR Sensor"=w256:dbl)
        "Left IR Sensor" <- w256
        n143 = Unbundle By Name(w261) -> ("Time up flag"=w262:bool)
        "Time up flag" <- w262
        n144 = Unbundle By Name(w263) -> ("Yaw"=w264:dbl, "Compass"=w258:dbl)
        n145 = Unbundle By Name(w265) -> ("y Stepper Position"=w267:u8, "z Stepper Position"=w266:u8)
        n146 = Unbundle By Name(w281) -> ("xDistance"=w278:dbl, "yDistance"=w279:dbl, "wDistance"=w280:dbl)
        n147 = Unbundle By Name(w269) -> ("Recognized Object"=w268:bool, "Object X coordinate"=w271:dbl, "Object Y coordinate"=w270:dbl)
        n148 = Unbundle By Name(w292) -> ("PING_A"=w284:u8, "PING_B"=w283:u8, "PING_C"=w282:u8, "PING_D"=w277:u8)
        n149 = case shown="39" w291 {
          tunnel: [w295 w301 w313 w322 w389 w402 w437 w489 w529 w571 w624 w670 w709 w768 w812 w851 w896 w939 w981 w1011 w1058 w1098] -> w290
          tunnel: w289 -> [w295 w304 w314 w325 w391 w403 w446 w487 w530 w577 w617 w673 w716 w758 w815 w857 w895 w934 w972 w1015 w1065 w1103]
          tunnel: [State_Type_Definitions."Idle" ("Enum") State_Type_Definitions."Idle" ("Enum") w309 w324 State_Type_Definitions."Shutdown" ("Enum") w404 w444 w490 w528 w572 w623 w671 w711 w767 w813 w858 w897 w940 w973 w1012 w1059 w1099] -> w288
          tunnel: w287 -> [_ _ w312 w328 _ w409 w440 w486 w537 w576 w621 w674 w715 w765 w810 w856 w893 w937 w980 w1019 w1064 w1106]
          tunnel: w286 -> [_ _ _ w327 _ w408 w439 w485 w536 w575 w620 w667 w714 w764 w809 w855 w892 w936 w978 w1014 w1063 w1105]
          tunnel: w285 -> [_ _ w311 w323 _ w407 w438 w484 w535 w574 w619 w666 w713 w766 w811 w854 w891 w935 w979 w1018 w1062 w1104]
          tunnel: w274 -> [_ _ _ _ _ w401 w445 w483 w532 w570 w622 w672 w717 w759 w816 w852 w894 w938 w976 w1017 w1057 w1102]
          tunnel: w284 -> [_ _ _ _ _ _ _ _ _ _ _ _ _ _ _ _ _ _ _ _ _ _]
          tunnel: w283 -> [_ _ _ _ _ _ _ w482 _ _ w613 w655 w707 _ w802 _ _ _ _ _ _ _]
          tunnel: w282 -> [_ _ _ _ _ _ _ w481 _ _ w614 w656 w708 _ w803 _ _ _ _ _ _ _]
          tunnel: w280 -> [_ _ _ _ _ _ _ _ w534 _ _ _ _ _ _ _ _ _ _ _ _ _]
          tunnel: w279 -> [_ _ _ _ _ w400 _ _ _ _ _ _ w712 _ _ _ _ _ _ _ _ _]
          tunnel: w278 -> [_ _ _ _ _ _ _ _ _ _ _ w661 _ _ _ _ _ _ _ _ _ _]
          tunnel: w277 -> [_ _ _ _ _ _ _ _ _ _ _ _ _ _ _ _ _ _ _ _ _ _]
          tunnel: [State_Type_Definitions."Idle" ("Enum") State_Type_Definitions."Idle" ("Enum") State_Type_Definitions."Idle" ("Enum") State_Type_Definitions."Idle" ("Enum") State_Type_Definitions."Shutdown" ("Enum") w397 w443 w488 w525 w569 w616 w669 w710 w769 w814 w850 w898 w941 w974 w1013 w1060 w1101] -> w273
          tunnel: w272 -> [_ _ w309 _ _ _ _ _ _ _ _ _ _ _ _ _ _ _ _ _ _ _]
          tunnel: w268 -> [_ _ _ _ _ _ _ _ _ _ _ _ _ _ _ _ w888 _ w975 _ _ _]
          tunnel: w271 -> [_ _ _ _ _ _ _ _ _ _ _ _ _ _ _ _ _ _ _ _ _ _]
          tunnel: w270 -> [_ _ _ _ _ _ _ _ _ _ _ _ _ _ _ _ _ _ _ _ _ _]
          tunnel: w267 -> [_ _ _ _ _ _ _ _ _ _ _ _ _ _ _ _ _ _ _ _ _ _]
          tunnel: w266 -> [_ _ _ _ _ _ w442 _ _ w567 _ _ _ w762 _ _ _ w933 _ w1016 _ _]
          tunnel: w264 -> [_ _ _ _ _ _ _ _ _ _ _ _ _ _ _ _ _ _ _ _ _ _]
          tunnel: w262 -> [_ _ _ _ _ _ _ _ _ _ _ _ _ _ _ w848 _ _ _ _ _ _]
          tunnel: w260 -> [w293 w299 w308 w320 w387 w396 w441 w480 w524 w568 w615 w665 w706 w757 w807 w849 w889 w930 w971 w1010 w1061 w1100]
          tunnel: [w293 w298 w308 w320 w387 w396 w441 w480 w524 w568 w615 w665 w706 w757 w807 w849 w889 w930 w971 w1010 w1061 w1100] -> w259
          tunnel: w258 -> [_ _ _ _ _ _ _ _ _ _ _ _ _ _ _ _ _ _ _ _ w1056 _]
          tunnel: [_ _ _ TRUE _ _ _ _ _ _ _ _ _ _ _ _ _ _ _ _ _ _] -> w257
          tunnel: w256 -> [_ _ _ _ _ _ _ _ _ _ _ _ _ _ _ _ _ _ _ _ _ _]
          frame 0 {
            # ">>> yStepper command>>>"
          }
          frame 1 {
            # ">>> yStepper command>>>"
            n150 = for {
              shift-right: [w307] -> w301
              shift-left: w304 -> [w306]
              tunnel: string[] ["INIT", "RESET ARM", "RESET FLAGS", "RESET YAW", "NAVX CALIBRATE"] -> [w305] mode=indexing
              n151 = Enqueue Element(queue=w306, element=w305) -> (queue out=w307:refnum<queue>)  [unwired: 2 in, 2 out]
            }
            n152 = Bundle By Name(cluster=w299, "yStepper desired"=u8 0) -> (w298:T9)
          }
          frame 3 {
            # ">>> yStepper command>>>"
            n153 = Flush Queue(queue=w312, error in (no error)=w311) -> ()  [unwired: 3 out]
            n154 = for {
              shift-right: [w318] -> w313
              shift-left: w314 -> [w317]
              tunnel: string[] ["STOP", "RESET ENCODERS", "RESET YAW", "RESET ARM", "RESET FLAGS", "DISPOSE BUFFERS", "CAM CLOSE"] -> [w316] mode=indexing
              n155 = Enqueue Element(queue=w317, element=w316) -> (queue out=w318:refnum<queue>)  [unwired: 2 in, 2 out]
            }
          }
          frame 4, Default {
            (unwired) TRUE ("Green LED")
            # ">>> yStepper command>>>"
            n156 = Dequeue Element(queue=w328, timeout in ms (-1)=w327, error in (no error)=w323) -> (element=w326:T7)  [unwired: 3 out]
            n157 = case shown="\"Start Task 9\"" w326 {
              tunnel: [w330 w337 w344 w351 w358 w365 w372 w374 w382] -> w322
              tunnel: w325 -> [w331 w338 w345 w352 w359 w366 w372 w375 w381]
              tunnel: [State_Type_Definitions."Task 1" ("Enum") State_Type_Definitions."Task 2:Raise Arm" ("Enum") State_Type_Definitions."Task 3" ("Enum") State_Type_Definitions."Task 4_A" ("Enum") State_Type_Definitions."Task 5_A" ("Enum") State_Type_Definitions."Task 6_A" ("Enum") State_Type_Definitions."Idle" ("Enum") State_Type_Definitions."Shutdown" ("Enum") State_Type_Definitions."Task 9A: Raise Arm" ("Enum")] -> w324
              frame "Start Task 1" {
                n158 = for {
                  shift-right: [w335] -> w330
                  shift-left: w331 -> [w334]
                  tunnel: string[] ["RESET ENCODERS", "RESET YAW", "FORWARD", "READ ENCODERS"] -> [w333] mode=indexing
                  n159 = Enqueue Element(queue=w334, element=w333) -> (queue out=w335:refnum<queue>)  [unwired: 2 in, 2 out]
                }
              }
              frame "Start Task 2" {
                n160 = for {
                  shift-right: [w342] -> w337
                  shift-left: w338 -> [w341]
                  tunnel: string[] ["RESET ENCODERS", "RESET YAW", "READ ULTRASONIC", "ARDUINO - ULTRASONIC"] -> [w340] mode=indexing
                  n161 = Enqueue Element(queue=w341, element=w340) -> (queue out=w342:refnum<queue>)  [unwired: 2 in, 2 out]
                }
              }
              frame "Start Task 3" {
                n162 = for {
                  shift-right: [w349] -> w344
                  shift-left: w345 -> [w348]
                  tunnel: string[] ["RESET ENCODERS", "READ ENCODERS", "R-ACW"] -> [w347] mode=indexing
                  n163 = Enqueue Element(queue=w348, element=w347) -> (queue out=w349:refnum<queue>)  [unwired: 2 in, 2 out]
                }
              }
              frame "Start Task 4" {
                n164 = for {
                  shift-right: [w356] -> w351
                  shift-left: w352 -> [w355]
                  tunnel: string[] ["RESET YAW", "RESET ENCODERS", "RESET ARM", "RESET FLAGS", "", ""] -> [w354] mode=indexing
                  n165 = Enqueue Element(queue=w355, element=w354) -> (queue out=w356:refnum<queue>)  [unwired: 2 in, 2 out]
                }
              }
              frame "Start Task 5" {
                n166 = for {
                  shift-right: [w363] -> w358
                  shift-left: w359 -> [w362]
                  tunnel: string[] ["RESET YAW", "RESET ENCODERS", "READ STEPPER VALUES", "Z STEPPER CAM HEIGHT", "", ""] -> [w361] mode=indexing
                  n167 = Enqueue Element(queue=w362, element=w361) -> (queue out=w363:refnum<queue>)  [unwired: 2 in, 2 out]
                }
              }
              frame "Start Task 6" {
                n168 = for {
                  shift-right: [w370] -> w365
                  shift-left: w366 -> [w369]
                  tunnel: string[] ["OPEN LOG CAM ", "", "", "", "", ""] -> [w368] mode=indexing
                  n169 = Enqueue Element(queue=w369, element=w368) -> (queue out=w370:refnum<queue>)  [unwired: 2 in, 2 out]
                }
              }
              frame "None", Default {
              }
              frame "Exit" {
                n170 = for {
                  shift-right: [w379] -> w374
                  shift-left: w375 -> [w378]
                  tunnel: string[] ["STOP", "RESET ENCODERS", "RESET YAW", "EXIT"] -> [w377] mode=indexing
                  n171 = Enqueue Element(queue=w378, element=w377) -> (queue out=w379:refnum<queue>)  [unwired: 2 in, 2 out]
                }
              }
              frame "Start Task 9" {
                n172 = for {
                  shift-right: [w386] -> w382
                  shift-left: w381 -> [w385]
                  tunnel: string[] ["RESET ENCODERS", "READ ENCODERS", "Z STEPPER CAM HEIGHT"] -> [w384] mode=indexing
                  n173 = Enqueue Element(queue=w385, element=w384) -> (queue out=w386:refnum<queue>)  [unwired: 2 in, 2 out]
                }
              }
            }
          }
          frame 5 {
            # ">>> yStepper command>>>"
            n174 = for {
              shift-right: [w395] -> w389
              shift-left: w391 -> [w394]
              tunnel: string[] ["INIT", "RESET ENCODERS", "RESET FLAGS", "CAM CLOSE", "DISPOSE BUFFERS", "EXIT", ""] -> [w393] mode=indexing
              n175 = Enqueue Element(queue=w394, element=w393) -> (queue out=w395:refnum<queue>)  [unwired: 2 in, 2 out]
            }
          }
          frame 6 {
            # ">>> yStepper command>>>"
            # "Use 250"
            n176 = Dequeue Element(queue=w409, timeout in ms (-1)=w408, error in (no error)=w407) -> (element=w406:T7)  [unwired: 3 out]
            n177 = Greater?(x=w400, y=250.0) -> (0:w398:bool)
            n178 = Or(x=w398, y=w401) -> (x .or. y?=w405:bool)
            n179 = case shown="\"None\", Default" w406 {
              tunnel: w405 -> [w412 _]
              tunnel: [w416 State_Type_Definitions."True Stop" ("Enum")] -> w404
              tunnel: w403 -> [w413 w431]
              tunnel: [w411 w430] -> w402
              tunnel: [State_Type_Definitions."Idle" ("Enum") State_Type_Definitions."Shutdown" ("Enum")] -> w397
              frame "None", Default {
                n180 = case shown="False" w412 {
                  tunnel: w413 -> [w419 w425]
                  tunnel: [w418 w423] -> w411
                  frame False {
                    n181 = for {
                      shift-right: [w421] -> w418
                      shift-left: w419 -> [w422]
                      tunnel: string[] ["READ ENCODERS", "READ NAVX", "FORWARD"] ("element") -> [w420] mode=indexing
                      n182 = Enqueue Element(queue=w422, element=w420) -> (queue out=w421:refnum<queue>)  [unwired: 2 in, 2 out]
                    }
                  }
                  frame True {
                    n183 = for {
                      shift-right: [w427] -> w423
                      shift-left: w425 -> [w428]
                      tunnel: string[] ["RESET YAW", "RESET ENCODERS", "STOP", ""] -> [w426] mode=indexing
                      n184 = Enqueue Element(queue=w428, element=w426) -> (queue out=w427:refnum<queue>)  [unwired: 2 in, 2 out]
                    }
                  }
                }
                n185 = Select(t=State_Type_Definitions."True Stop" ("Enum"), s=w412, f=State_Type_Definitions."Task 1" ("Enum")) -> (s? t:f=w416:u16)
              }
              frame "Exit" {
                n186 = for {
                  shift-right: [w435] -> w430
                  shift-left: w431 -> [w436]
                  tunnel: string[] ["STOP", "RESET ENCODERS", "RESET YAW", ""] -> [w434] mode=indexing
                  n187 = Enqueue Element(queue=w436, element=w434) -> (queue out=w435:refnum<queue>)  [unwired: 2 in, 2 out]
                }
              }
            }
          }
          frame 8 {
            # ">> Stepper height reeached >>"
            # ">>> yStepper command>>>"
            # ">> Manual override >>"
            n188 = Dequeue Element(queue=w440, timeout in ms (-1)=w439, error in (no error)=w438) -> (element=w449:T7)  [unwired: 3 out]
            n189 = Equal?(x=w442, y=u8 80) -> (x = y?=w447:bool)
            n190 = case shown="\"None\", Default" w449 {
              tunnel: [w460 State_Type_Definitions."True Stop" ("Enum")] -> w444
              tunnel: [w458 w475] -> w437
              tunnel: w446 -> [w457 _]
              tunnel: w445 -> [w451 _]
              tunnel: [State_Type_Definitions."Idle" ("Enum") State_Type_Definitions."Shutdown" ("Enum")] -> w443
              tunnel: w447 -> [w450 _]
              frame "None", Default {
                # ">> WIill proceed to part ii if not manual override >>"
                # ">>If ENABLE or Trigger is set to true>>"
                n191 = Or(x=w450, y=w451) -> (x .or. y?=w452:bool)
                n192 = case shown="True" w450 {
                  tunnel: [w463 w469] -> w458
                  tunnel: w457 -> [w462 w468]
                  frame False {
                    n193 = for {
                      shift-right: [w465] -> w463
                      shift-left: w462 -> [w466]
                      tunnel: string[] ["Z STEPPER CAM HEIGHT", "READ STEPPER VALUES"] ("element") -> [w464] mode=indexing
                      n194 = Enqueue Element(queue=w466, element=w464) -> (queue out=w465:refnum<queue>)  [unwired: 2 in, 2 out]
                    }
                  }
                  frame True {
                    n195 = for {
                      shift-right: [w471] -> w469
                      shift-left: w468 -> [w472]
                      tunnel: string[] ["ARDUINO - ULTRASONIC", "READ ULTRASONIC", "", "", "", ""] -> [w470] mode=indexing
                      n196 = Enqueue Element(queue=w472, element=w470) -> (queue out=w471:refnum<queue>)  [unwired: 2 in, 2 out]
                    }
                  }
                }
                n197 = Select(t=State_Type_Definitions."True Stop" ("Enum"), s=w451, f=State_Type_Definitions."Task 2:Sensor Mode" ("Enum")) -> (s? t:f=w454:T6)
                n198 = Select(t=w454, s=w452, f=State_Type_Definitions."Task 2:Raise Arm" ("Enum")) -> (s? t:f=w460:T6)
              }
              frame "Exit" {
                n199 = for {
                  shift-right: [w478] -> w475
                  shift-left: _ -> [w479]
                  tunnel: string[] ["STOP", "RESET ENCODERS", "RESET YAW", ""] -> [w477] mode=indexing
                  n200 = Enqueue Element(queue=w479, element=w477) -> (queue out=w478:refnum<queue>)  [unwired: 2 in, 2 out]
                }
              }
            }
          }
          frame 9 {
            w494 = u8 30 ("y")
            # ">>> yStepper command>>>"
            # ">>Object detected>>"
            n201 = Dequeue Element(queue=w486, timeout in ms (-1)=w485, error in (no error)=w484) -> (element=w495:T7)  [unwired: 3 out]
            n202 = Less?(x=w482, y=w494) -> (x < y?=w493:bool)
            n203 = Less?(x=w481, y=w494) -> (x < y?=w492:bool)
            n204 = Or(x=w493, y=w492) -> (x .or. y?=w491:bool)
            "Obstacle detected" <- w491
            n205 = case shown="\"None\", Default" w495 {
              tunnel: w491 -> [w499 _]
              tunnel: [w501 State_Type_Definitions."True Stop" ("Enum")] -> w490
              tunnel: w483 -> [w500 _]
              tunnel: w487 -> [w498 w518]
              tunnel: [w497 w519] -> w489
              tunnel: [State_Type_Definitions."Idle" ("Enum") State_Type_Definitions."Shutdown" ("Enum")] -> w488
              frame "None", Default {
                n206 = case shown="False" w499 {
                  tunnel: w498 -> [w505 w512]
                  tunnel: [w506 w511] -> w497
                  frame False {
                    n207 = for {
                      tunnel: string[] ["READ ULTRASONIC", "STOP"] ("element") -> [w507] mode=indexing
                      shift-right: [w509] -> w506
                      shift-left: w505 -> [w508]
                      n208 = Enqueue Element(queue=w508, element=w507) -> (queue out=w509:refnum<queue>)  [unwired: 2 in, 2 out]
                    }
                  }
                  frame True {
                    n209 = for {
                      shift-right: [w514] -> w511
                      shift-left: w512 -> [w515]
                      tunnel: string[] ["REVERSE", "READ ULTRASONIC", "READ NAVX"] -> [w513] mode=indexing
                      n210 = Enqueue Element(queue=w515, element=w513) -> (queue out=w514:refnum<queue>)  [unwired: 2 in, 2 out]
                    }
                  }
                }
                n211 = Select(t=State_Type_Definitions."True Stop" ("Enum"), s=w500, f=State_Type_Definitions."Task 2:Sensor Mode" ("Enum")) -> (s? t:f=w501:T6)
              }
              frame "Exit" {
                n212 = for {
                  shift-right: [w522] -> w519
                  shift-left: w518 -> [w523]
                  tunnel: string[] ["STOP", "RESET ENCODERS", "RESET YAW", "ARDUINO MODE 0"] -> [w521] mode=indexing
                  n213 = Enqueue Element(queue=w523, element=w521) -> (queue out=w522:refnum<queue>)  [unwired: 2 in, 2 out]
                }
              }
            }
          }
          frame 11 {
            # ">>> yStepper command>>>"
            n214 = Dequeue Element(queue=w537, timeout in ms (-1)=w536, error in (no error)=w535) -> (element=w526:T7)  [unwired: 3 out]
            n215 = Greater?(x=w534, y=160.0) -> (0:w531:bool)
            n216 = Or(x=w531, y=w532) -> (x .or. y?=w527:bool)
            n217 = case shown="\"None\", Default" w526 {
              tunnel: w527 -> [w540 _]
              tunnel: [w544 State_Type_Definitions."True Stop" ("Enum")] -> w528
              tunnel: w530 -> [w541 w560]
              tunnel: [w539 w559] -> w529
              tunnel: [State_Type_Definitions."Idle" ("Enum") State_Type_Definitions."Shutdown" ("Enum")] -> w525
              frame "None", Default {
                n218 = case shown="False" w540 {
                  tunnel: w541 -> [w547 w553]
                  tunnel: [w546 w551] -> w539
                  frame False {
                    n219 = for {
                      shift-right: [w549] -> w546
                      shift-left: w547 -> [w550]
                      tunnel: string[] ["READ ENCODERS", "R-ACW"] ("element") -> [w548] mode=indexing
                      n220 = Enqueue Element(queue=w550, element=w548) -> (queue out=w549:refnum<queue>)  [unwired: 2 in, 2 out]
                    }
                  }
                  frame True {
                    n221 = for {
                      shift-right: [w555] -> w551
                      shift-left: w553 -> [w556]
                      tunnel: string[] ["RESET YAW", "RESET ENCODERS", "STOP", "ARDUINO MODE 0"] -> [w554] mode=indexing
                      n222 = Enqueue Element(queue=w556, element=w554) -> (queue out=w555:refnum<queue>)  [unwired: 2 in, 2 out]
                    }
                  }
                }
                n223 = Select(t=State_Type_Definitions."True Stop" ("Enum"), s=w540, f=State_Type_Definitions."Task 3" ("Enum")) -> (s? t:f=w544:T6)
              }
              frame "Exit" {
                n224 = for {
                  shift-right: [w563] -> w559
                  shift-left: w560 -> [w564]
                  tunnel: string[] ["STOP", "RESET ENCODERS", "RESET YAW", ""] -> [w562] mode=indexing
                  n225 = Enqueue Element(queue=w564, element=w562) -> (queue out=w563:refnum<queue>)  [unwired: 2 in, 2 out]
                }
              }
            }
          }
          frame 12 {
            # ">> Stepper height reeached >>"
            # ">>> yStepper command>>>"
            # ">> Manual override >>"
            n226 = Dequeue Element(queue=w576, timeout in ms (-1)=w575, error in (no error)=w574) -> (element=w573:T7)  [unwired: 3 out]
            n227 = Equal?(x=w567, y=u8 80) -> (x = y?=w565:bool)
            n228 = case shown="\"Exit\"" w573 {
              tunnel: [w588 State_Type_Definitions."True Stop" ("Enum")] -> w572
              tunnel: [w586 w604] -> w571
              tunnel: w577 -> [w585 w601]
              tunnel: w570 -> [w579 _]
              tunnel: [State_Type_Definitions."Idle" ("Enum") State_Type_Definitions."Shutdown" ("Enum")] -> w569
              tunnel: w565 -> [w578 _]
              frame "None", Default {
                # ">> WIill proceed to part ii if not manual override >>"
                # ">>If ENABLE or Trigger is set to true>>"
                n229 = Or(x=w578, y=w579) -> (x .or. y?=w580:bool)
                n230 = case shown="False" w578 {
                  tunnel: [w591 w597] -> w586
                  tunnel: w585 -> [w590 w596]
                  frame False {
                    n231 = for {
                      shift-right: [w593] -> w591
                      shift-left: w590 -> [w594]
                      tunnel: string[] ["Z STEPPER CAM HEIGHT", "READ STEPPER VALUES"] ("element") -> [w592] mode=indexing
                      n232 = Enqueue Element(queue=w594, element=w592) -> (queue out=w593:refnum<queue>)  [unwired: 2 in, 2 out]
                    }
                  }
                  frame True {
                    n233 = for {
                      shift-right: [w599] -> w597
                      shift-left: w596 -> [w600]
                      tunnel: string[] ["ARDUINO - ULTRASONIC", "READ ULTRASONIC", "FORWARD", "", "", ""] -> [w598] mode=indexing
                      n234 = Enqueue Element(queue=w600, element=w598) -> (queue out=w599:refnum<queue>)  [unwired: 2 in, 2 out]
                    }
                  }
                }
                n235 = Select(t=State_Type_Definitions."True Stop" ("Enum"), s=w579, f=State_Type_Definitions."Task 4_B" ("Enum")) -> (s? t:f=w582:T6)
                n236 = Select(t=w582, s=w580, f=State_Type_Definitions."Task 4_A" ("Enum")) -> (s? t:f=w588:T6)
              }
              frame "Exit" {
                n237 = for {
                  shift-right: [w607] -> w604
                  shift-left: w601 -> [w608]
                  tunnel: string[] ["STOP", "RESET ENCODERS", "RESET YAW", ""] -> [w606] mode=indexing
                  n238 = Enqueue Element(queue=w608, element=w606) -> (queue out=w607:refnum<queue>)  [unwired: 2 in, 2 out]
                }
              }
            }
          }
          frame 13 {
            w612 = u8 20
            # ">> Path blocked >>"
            # ">>> yStepper command>>>"
            # ">> Manual override >>"
            n239 = Dequeue Element(queue=w621, timeout in ms (-1)=w620, error in (no error)=w619) -> (element=w618:T7)  [unwired: 3 out]
            n240 = Less?(x=w614, y=w612) -> (x < y?=w609:bool)
            n241 = Less?(x=w613, y=w612) -> (x < y?=w610:bool)
            n242 = And(x=w610, y=w609) -> (x .and. y?=w611:bool)
            n243 = case shown="\"None\", Default" w618 {
              tunnel: [w635 State_Type_Definitions."True Stop" ("Enum")] -> w623
              tunnel: [w633 w650] -> w624
              tunnel: w617 -> [w632 _]
              tunnel: w622 -> [w626 _]
              tunnel: [State_Type_Definitions."Idle" ("Enum") State_Type_Definitions."Shutdown" ("Enum")] -> w616
              tunnel: w611 -> [w625 _]
              frame "None", Default {
                # ">> Manual override forces program to true stop >>"
                # ">>If ENABLE or Trigger is set to true>>"
                n244 = Or(x=w625, y=w626) -> (x .or. y?=w631:bool)
                n245 = case shown="False" w625 {
                  tunnel: [w638 w643] -> w633
                  tunnel: w632 -> [w637 w642]
                  frame False {
                    n246 = for {
                      shift-right: [w640] -> w638
                      shift-left: w637 -> [w641]
                      tunnel: string[] ["FORWARD", "READ ULTRASONIC", "READ NAVX"] ("element") -> [w639] mode=indexing
                      n247 = Enqueue Element(queue=w641, element=w639) -> (queue out=w640:refnum<queue>)  [unwired: 2 in, 2 out]
                    }
                  }
                  frame True {
                    n248 = for {
                      shift-right: [w646] -> w643
                      shift-left: w642 -> [w647]
                      tunnel: string[] ["STOP", "RESET YAW", "RESET ENCODERS", "RESET FLAGS"] -> [w645] mode=indexing
                      n249 = Enqueue Element(queue=w647, element=w645) -> (queue out=w646:refnum<queue>)  [unwired: 2 in, 2 out]
                    }
                  }
                }
                n250 = Select(t=State_Type_Definitions."True Stop" ("Enum"), s=w626, f=State_Type_Definitions."Task 4_C" ("Enum")) -> (s? t:f=w628:T6)
                n251 = Select(t=w628, s=w631, f=State_Type_Definitions."Task 4_B" ("Enum")) -> (s? t:f=w635:T6)
              }
              frame "Exit" {
                n252 = for {
                  shift-right: [w653] -> w650
                  shift-left: _ -> [w654]
                  tunnel: string[] ["STOP", "RESET ENCODERS", "RESET YAW", ""] -> [w652] mode=indexing
                  n253 = Enqueue Element(queue=w654, element=w652) -> (queue out=w653:refnum<queue>)  [unwired: 2 in, 2 out]
                }
              }
            }
          }
          frame 14 {
            w664 = u8 20
            # ">> xDistance travelled>>"
            # ">> Path NOT blocked >>"
            # ">>> yStepper command>>>"
            # ">> Manual override >>"
            n254 = Dequeue Element(queue=w674, timeout in ms (-1)=w667, error in (no error)=w666) -> (element=w668:T7)  [unwired: 3 out]
            n255 = Greater?(x=w656, y=w664) -> (0:w662:bool)
            n256 = Greater?(x=w661, y=80.0) -> (0:w659:bool)
            n257 = Greater?(x=w655, y=w664) -> (0:w663:bool)
            n258 = And(x=w663, y=w662) -> (x .and. y?=w658:bool)
            n259 = And(x=w659, y=w658) -> (x .and. y?=w657:bool)
            n260 = case shown="\"None\", Default" w668 {
              tunnel: [w685 State_Type_Definitions."True Stop" ("Enum")] -> w671
              tunnel: [w683 w701] -> w670
              tunnel: w673 -> [w682 w698]
              tunnel: w672 -> [w676 _]
              tunnel: [State_Type_Definitions."Idle" ("t") State_Type_Definitions."Shutdown" ("Enum")] -> w669
              tunnel: w657 -> [w675 _]
              frame "None", Default {
                # ">> Manual override forces program to true stop >>"
                # ">>If ENABLE or Trigger is set to true>>"
                n261 = Or(x=w675, y=w676) -> (x .or. y?=w681:bool)
                n262 = case shown="False" w675 {
                  tunnel: [w688 w693] -> w683
                  tunnel: w682 -> [w686 w692]
                  frame False {
                    n263 = for {
                      shift-right: [w690] -> w688
                      shift-left: w686 -> [w691]
                      tunnel: string[] ["RIGHT", "READ NAVX", "READ ENCODERS", "READ ULTRASONIC"] ("element") -> [w689] mode=indexing
                      n264 = Enqueue Element(queue=w691, element=w689) -> (queue out=w690:refnum<queue>)  [unwired: 2 in, 2 out]
                    }
                  }
                  frame True {
                    n265 = for {
                      shift-right: [w696] -> w693
                      shift-left: w692 -> [w697]
                      tunnel: string[] ["STOP", "RESET YAW", "RESET ENCODERS", "ARDUINO - ULTRASONIC"] -> [w695] mode=indexing
                      n266 = Enqueue Element(queue=w697, element=w695) -> (queue out=w696:refnum<queue>)  [unwired: 2 in, 2 out]
                    }
                  }
                }
                n267 = Select(t=State_Type_Definitions."True Stop" ("Enum"), s=w676, f=State_Type_Definitions."Task 4_D" ("Enum")) -> (s? t:f=w677:T6)
                n268 = Select(t=w677, s=w681, f=State_Type_Definitions."Task 4_C" ("Enum")) -> (s? t:f=w685:T6)
              }
              frame "Exit" {
                n269 = for {
                  shift-right: [w704] -> w701
                  shift-left: w698 -> [w705]
                  tunnel: string[] ["STOP", "RESET ENCODERS", "RESET YAW", ""] -> [w703] mode=indexing
                  n270 = Enqueue Element(queue=w705, element=w703) -> (queue out=w704:refnum<queue>)  [unwired: 2 in, 2 out]
                }
              }
            }
          }
          frame 15 {
            w724 = u8 20
            # ">> yDistance travelled>>"
            # ">> Path blocked >>"
            # ">>> yStepper command>>>"
            # ">> Manual override >>"
            n271 = Dequeue Element(queue=w715, timeout in ms (-1)=w714, error in (no error)=w713) -> (element=w725:T7)  [unwired: 3 out]
            n272 = Less?(x=w708, y=w724) -> (x < y?=w722:bool)
            n273 = Greater?(x=w712, y=200.0) -> (0:w720:bool)
            n274 = Less?(x=w707, y=w724) -> (x < y?=w723:bool)
            n275 = And(x=w723, y=w722) -> (x .and. y?=w719:bool)
            n276 = Or(x=w720, y=w719) -> (x .or. y?=w718:bool)
            n277 = case shown="\"None\", Default" w725 {
              tunnel: [w736 State_Type_Definitions."True Stop" ("Enum")] -> w711
              tunnel: [w734 w752] -> w709
              tunnel: w716 -> [w733 w749]
              tunnel: w717 -> [w727 _]
              tunnel: [State_Type_Definitions."Idle" ("t") State_Type_Definitions."Shutdown" ("Enum")] -> w710
              tunnel: w718 -> [w726 _]
              frame "None", Default {
                # ">> Manual override forces program to true stop >>"
                # ">>If ENABLE or Trigger is set to true>>"
                n278 = Or(x=w726, y=w727) -> (x .or. y?=w732:bool)
                n279 = case shown="True" w726 {
                  tunnel: [w739 w744] -> w734
                  tunnel: w733 -> [w737 w743]
                  frame False {
                    n280 = for {
                      shift-right: [w741] -> w739
                      shift-left: w737 -> [w742]
                      tunnel: string[] ["FORWARD", "READ NAVX", "READ ENCODERS", "READ ULTRASONIC"] ("element") -> [w740] mode=indexing
                      n281 = Enqueue Element(queue=w742, element=w740) -> (queue out=w741:refnum<queue>)  [unwired: 2 in, 2 out]
                    }
                  }
                  frame True {
                    n282 = for {
                      shift-right: [w747] -> w744
                      shift-left: w743 -> [w748]
                      tunnel: string[] ["STOP", "RESET YAW", "RESET ENCODERS", "RESET FLAGS"] -> [w746] mode=indexing
                      n283 = Enqueue Element(queue=w748, element=w746) -> (queue out=w747:refnum<queue>)  [unwired: 2 in, 2 out]
                    }
                  }
                }
                n284 = Select(t=State_Type_Definitions."True Stop" ("Enum"), s=w727, f=State_Type_Definitions."True Stop" ("Enum")) -> (s? t:f=w728:T6)
                n285 = Select(t=w728, s=w732, f=State_Type_Definitions."Task 4_D" ("Enum")) -> (s? t:f=w736:T6)
              }
              frame "Exit" {
                n286 = for {
                  shift-right: [w755] -> w752
                  shift-left: w749 -> [w756]
                  tunnel: string[] ["STOP", "RESET ENCODERS", "RESET YAW", ""] -> [w754] mode=indexing
                  n287 = Enqueue Element(queue=w756, element=w754) -> (queue out=w755:refnum<queue>)  [unwired: 2 in, 2 out]
                }
              }
            }
          }
          frame 14 {
            # ">>> yStepper command>>>"
            # ">> Manual override >>"
            n288 = Dequeue Element(queue=w765, timeout in ms (-1)=w764, error in (no error)=w766) -> (element=w763:T7)  [unwired: 3 out]
            n289 = Equal?(x=w762, y=u8 80) -> (x = y?=w760:bool)
            n290 = case shown="\"None\", Default" w763 {
              tunnel: [w776 State_Type_Definitions."True Stop" ("Enum")] -> w767
              tunnel: [w779 w796] -> w768
              tunnel: [State_Type_Definitions."Idle" ("Enum") State_Type_Definitions."Shutdown" ("Enum")] -> w769
              tunnel: w760 -> [w775 _]
              tunnel: w759 -> [w774 _]
              tunnel: w758 -> [w770 w793]
              frame "None", Default {
                # "Stays in Task 5_A until stepper reaches desired \nheight"
                # "T: Go back to idle, F: Continue with task\""
                # ">> Manual override >>"
                n291 = case shown="True" w775 {
                  tunnel: [w783 w789] -> w779
                  tunnel: w770 -> [w781 w787]
                  frame False {
                    n292 = for {
                      tunnel: string[] ["Z STEPPER CAM HEIGHT", "READ STEPPER VALUES"] ("element") -> [w784] mode=indexing
                      shift-right: [w786] -> w783
                      shift-left: w781 -> [w785]
                      n293 = Enqueue Element(queue=w785, element=w784) -> (queue out=w786:refnum<queue>)  [unwired: 2 in, 2 out]
                    }
                  }
                  frame True {
                    n294 = for {
                      shift-right: [w791] -> w789
                      shift-left: w787 -> [w792]
                      tunnel: string[] ["ARDUINO - ULTRASONIC", "READ ULTRASONIC", ""] -> [w790] mode=indexing
                      n295 = Enqueue Element(queue=w792, element=w790) -> (queue out=w791:refnum<queue>)  [unwired: 2 in, 2 out]
                    }
                  }
                }
                n296 = Or(x=w775, y=w774) -> (x .or. y?=w777:bool)
                n297 = Select(t=State_Type_Definitions."True Stop" ("Enum"), s=w774, f=State_Type_Definitions."Task 5 _B" ("Enum")) -> (s? t:f=w771:u16)
                n298 = Select(t=w771, s=w777, f=State_Type_Definitions."Task 5_A" ("Enum")) -> (s? t:f=w776:u16)
              }
              frame "Exit" {
                n299 = for {
                  shift-right: [w799] -> w796
                  shift-left: w793 -> [w800]
                  tunnel: string[] ["STOP", "RESET ENCODERS", "RESET YAW", "ARDUINO MODE 0"] -> [w798] mode=indexing
                  n300 = Enqueue Element(queue=w800, element=w798) -> (queue out=w799:refnum<queue>)  [unwired: 2 in, 2 out]
                }
              }
            }
          }
          frame 15 {
            w806 = u8 20 ("y")
            # ">>> yStepper command>>>"
            n301 = Less?(x=w803, y=w806) -> (x < y?=w804:bool)
            n302 = Dequeue Element(queue=w810, timeout in ms (-1)=w809, error in (no error)=w811) -> (element=w808:T7)  [unwired: 3 out]
            n303 = Less?(x=w802, y=w806) -> (x < y?=w805:bool)
            n304 = And(x=w805, y=w804) -> (x .and. y?=w801:bool)
            n305 = case shown="\"Exit\"" w808 {
              tunnel: [w823 State_Type_Definitions."True Stop" ("Enum")] -> w813
              tunnel: [w826 w843] -> w812
              tunnel: [State_Type_Definitions."Idle" ("Enum") State_Type_Definitions."Shutdown" ("Enum")] -> w814
              tunnel: w816 -> [w822 _]
              tunnel: w815 -> [w818 w840]
              tunnel: w801 -> [w817 _]
              frame "None", Default {
                # "Stays in Task 5_B to capture image over 5 seconds"
                # "T: Go back to idle, F: Continue with task\""
                # ">> Manual override >>"
                n306 = case shown="False" w817 {
                  tunnel: [w830 w836] -> w826
                  tunnel: w818 -> [w828 w834]
                  frame False {
                    n307 = for {
                      tunnel: string[] ["FORWARD", "READ ULTRASONIC", "READ NAVX"] ("element") -> [w831] mode=indexing
                      shift-right: [w833] -> w830
                      shift-left: w828 -> [w832]
                      n308 = Enqueue Element(queue=w832, element=w831) -> (queue out=w833:refnum<queue>)  [unwired: 2 in, 2 out]
                    }
                  }
                  frame True {
                    n309 = for {
                      shift-right: [w838] -> w836
                      shift-left: w834 -> [w839]
                      tunnel: string[] ["STOP", "RESET ENCODERS", "OPEN LOG CAM", "SET TIMER"] -> [w837] mode=indexing
                      n310 = Enqueue Element(queue=w839, element=w837) -> (queue out=w838:refnum<queue>)  [unwired: 2 in, 2 out]
                    }
                  }
                }
                n311 = Or(x=w817, y=w822) -> (x .or. y?=w824:bool)
                n312 = Select(t=State_Type_Definitions."True Stop" ("Enum"), s=w822, f=State_Type_Definitions."Task 5_C" ("Enum")) -> (s? t:f=w819:u16)
                n313 = Select(t=w819, s=w824, f=State_Type_Definitions."Task 5 _B" ("Enum")) -> (s? t:f=w823:u16)
              }
              frame "Exit" {
                n314 = for {
                  shift-right: [w846] -> w843
                  shift-left: w840 -> [w847]
                  tunnel: string[] ["STOP", "RESET ENCODERS", "RESET YAW", "ARDUINO MODE 0"] -> [w845] mode=indexing
                  n315 = Enqueue Element(queue=w847, element=w845) -> (queue out=w846:refnum<queue>)  [unwired: 2 in, 2 out]
                }
              }
            }
          }
          frame 16 {
            # ">>> yStepper command>>>"
            # ">> Manual override >>"
            n316 = Dequeue Element(queue=w856, timeout in ms (-1)=w855, error in (no error)=w854) -> (element=w853:T7)  [unwired: 3 out]
            n317 = case shown="\"None\", Default" w853 {
              tunnel: [w863 State_Type_Definitions."True Stop" ("Enum")] -> w858
              tunnel: [w866 w883] -> w851
              tunnel: [State_Type_Definitions."Idle" ("Enum") State_Type_Definitions."Shutdown" ("Enum")] -> w850
              tunnel: w852 -> [w860 _]
              tunnel: w857 -> [w862 w880]
              tunnel: w848 -> [w859 _]
              frame "None", Default {
                # ">> Is time up? >>"
                # "Determines if object is in range to pick up"
                # ">> Manual override >>"
                n318 = case shown="False" w859 {
                  tunnel: [w870 w876] -> w866
                  tunnel: w862 -> [w868 w874]
                  frame False {
                    n319 = for {
                      tunnel: string[] ["CAM ACQ", "START TIMER"] ("element") -> [w871] mode=indexing
                      shift-right: [w873] -> w870
                      shift-left: w868 -> [w872]
                      n320 = Enqueue Element(queue=w872, element=w871) -> (queue out=w873:refnum<queue>)  [unwired: 2 in, 2 out]
                    }
                  }
                  frame True {
                    n321 = for {
                      shift-right: [w878] -> w876
                      shift-left: w874 -> [w879]
                      tunnel: string[] ["CAM CLOSE", "PROCESS IMAGE"] -> [w877] mode=indexing
                      n322 = Enqueue Element(queue=w879, element=w877) -> (queue out=w878:refnum<queue>)  [unwired: 2 in, 2 out]
                    }
                  }
                }
                n323 = Or(x=w859, y=w860) -> (x .or. y?=w864:bool)
                n324 = Select(t=State_Type_Definitions."Task 5_D" ("Enum"), s=w864, f=State_Type_Definitions."Task 5_D" ("Enum")) -> (s? t:f=w863:T24)
              }
              frame "Exit" {
                n325 = for {
                  shift-right: [w886] -> w883
                  shift-left: w880 -> [w887]
                  tunnel: string[] ["STOP", "RESET ENCODERS", "RESET YAW", "ARDUINO MODE 0"] -> [w885] mode=indexing
                  n326 = Enqueue Element(queue=w887, element=w885) -> (queue out=w886:refnum<queue>)  [unwired: 2 in, 2 out]
                }
              }
            }
          }
          frame 17 {
            # ">>> yStepper command>>>"
            n327 = Dequeue Element(queue=w893, timeout in ms (-1)=w892, error in (no error)=w891) -> (element=w890:T7)  [unwired: 3 out]
            n328 = case shown="\"None\", Default" w890 {
              tunnel: [w905 State_Type_Definitions."True Stop" ("Enum")] -> w897
              tunnel: [w908 w925] -> w896
              tunnel: [State_Type_Definitions."Idle" ("Enum") State_Type_Definitions."Shutdown" ("Enum")] -> w898
              tunnel: w894 -> [w904 _]
              tunnel: w895 -> [w900 w922]
              tunnel: w888 -> [w899 _]
              frame "None", Default {
                # ">> T: Breaks out of state loop; F: Stays in loop>>"
                # ">> Manual override >>"
                # ">> Checks if object is detected>>"
                # "Stays in Task 5D until the object is detected"
                # "T: Go back to idle, F: Continue with task\""
                # ">> Manual override >>"
                n329 = case shown="False" w899 {
                  tunnel: [w912 w918] -> w908
                  tunnel: w900 -> [w910 w916]
                  frame False {
                    n330 = for {
                      tunnel: string[] ["PROCESS IMAGE", "", ""] ("element") -> [w913] mode=indexing
                      shift-right: [w915] -> w912
                      shift-left: w910 -> [w914]
                      n331 = Enqueue Element(queue=w914, element=w913) -> (queue out=w915:refnum<queue>)  [unwired: 2 in, 2 out]
                    }
                  }
                  frame True {
                    n332 = for {
                      shift-right: [w920] -> w918
                      shift-left: w916 -> [w921]
                      tunnel: string[] ["DISPOSE BUFFERS", "CAM CLOSE", ""] -> [w919] mode=indexing
                      n333 = Enqueue Element(queue=w921, element=w919) -> (queue out=w920:refnum<queue>)  [unwired: 2 in, 2 out]
                    }
                  }
                }
                n334 = Or(x=w899, y=w904) -> (x .or. y?=w906:bool)
                n335 = Select(t=State_Type_Definitions."True Stop" ("Enum"), s=w904, f=State_Type_Definitions."True Stop" ("Enum")) -> (s? t:f=w901:T6)
                n336 = Select(t=w901, s=w906, f=State_Type_Definitions."Task 5_D" ("Enum")) -> (s? t:f=w905:u16)
              }
              frame "Exit" {
                n337 = for {
                  shift-right: [w928] -> w925
                  shift-left: w922 -> [w929]
                  tunnel: string[] ["STOP", "RESET ENCODERS", "RESET YAW", "ARDUINO MODE 0"] -> [w927] mode=indexing
                  n338 = Enqueue Element(queue=w929, element=w927) -> (queue out=w928:refnum<queue>)  [unwired: 2 in, 2 out]
                }
              }
            }
          }
          frame 24 {
            # ">>> yStepper command>>>"
            n339 = Dequeue Element(queue=w937, timeout in ms (-1)=w936, error in (no error)=w935) -> (element=w942:T7)  [unwired: 3 out]
            n340 = Equal?(x=w933, y=u8 80) -> (x = y?=w932:bool)
            n341 = case shown="\"None\", Default" w942 {
              tunnel: [w949 State_Type_Definitions."True Stop" ("Enum")] -> w940
              tunnel: [w948 w966] -> w939
              tunnel: [State_Type_Definitions."Idle" ("Enum") State_Type_Definitions."Shutdown" ("Enum")] -> w941
              tunnel: w938 -> [w944 _]
              tunnel: w934 -> [w946 _]
              tunnel: w932 -> [w943 _]
              frame "None", Default {
                n342 = case shown="False" w943 {
                  tunnel: [w954 w960] -> w948
                  tunnel: w946 -> [w952 w958]
                  frame False {
                    n343 = for {
                      tunnel: string[] ["Z STEPPER CAM HEIGHT", "READ STEPPER VALUES"] ("element") -> [w955] mode=indexing
                      shift-right: [w957] -> w954
                      shift-left: w952 -> [w956]
                      n344 = Enqueue Element(queue=w956, element=w955) -> (queue out=w957:refnum<queue>)  [unwired: 2 in, 2 out]
                    }
                  }
                  frame True {
                    n345 = for {
                      shift-right: [w962] -> w960
                      shift-left: w958 -> [w963]
                      tunnel: string[] ["CAM ACQ", "OPEN LOG CAM"] -> [w961] mode=indexing
                      n346 = Enqueue Element(queue=w963, element=w961) -> (queue out=w962:refnum<queue>)  [unwired: 2 in, 2 out]
                    }
                  }
                }
                n347 = Or(x=w943, y=w944) -> (x .or. y?=w945:bool)
                n348 = Select(t=State_Type_Definitions."Task 6_B" ("Enum"), s=w945, f=State_Type_Definitions."Task 6_A" ("Enum")) -> (s? t:f=w949:T6)
              }
              frame "Exit" {
                n349 = for {
                  shift-right: [w969] -> w966
                  shift-left: _ -> [w970]
                  tunnel: string[] ["STOP", "RESET ENCODERS", "RESET YAW", "ARDUINO MODE 0"] -> [w968] mode=indexing
                  n350 = Enqueue Element(queue=w970, element=w968) -> (queue out=w969:refnum<queue>)  [unwired: 2 in, 2 out]
                }
              }
            }
          }
          frame 25 {
            # ">>> yStepper command>>>"
            n351 = Dequeue Element(queue=w980, timeout in ms (-1)=w978, error in (no error)=w979) -> (element=w977:T7)  [unwired: 3 out]
            n352 = case shown="\"None\", Default" w977 {
              tunnel: [w987 State_Type_Definitions."True Stop" ("Enum")] -> w973
              tunnel: [w986 w1005] -> w981
              tunnel: [State_Type_Definitions."Idle" ("Enum") State_Type_Definitions."Shutdown" ("Enum")] -> w974
              tunnel: w976 -> [w982 _]
              tunnel: w975 -> [w984 _]
              tunnel: w972 -> [w983 w1002]
              frame "None", Default {
                # ">> Manual override >>"
                n353 = case shown="True" w984 {
                  tunnel: [w992 w998] -> w986
                  tunnel: w983 -> [w991 w996]
                  frame False {
                    n354 = for {
                      shift-right: [w995] -> w992
                      shift-left: w991 -> [w994]
                      tunnel: string[] ["CAM ACQ", "PROCESS IMAGE", "OPEN CLAW"] -> [w993] mode=indexing
                      n355 = Enqueue Element(queue=w994, element=w993) -> (queue out=w995:refnum<queue>)  [unwired: 2 in, 2 out]
                    }
                  }
                  frame True {
                    n356 = for {
                      shift-right: [w1000] -> w998
                      shift-left: w996 -> [w1001]
                      tunnel: string[] ["CAM ACQ", "PROCESS IMAGE", "CLOSE CLAW"] -> [w999] mode=indexing
                      n357 = Enqueue Element(queue=w1001, element=w999) -> (queue out=w1000:refnum<queue>)  [unwired: 2 in, 2 out]
                    }
                  }
                }
                n358 = Select(t=State_Type_Definitions."True Stop" ("Enum"), s=w982, f=State_Type_Definitions."Task 6_B" ("Enum")) -> (s? t:f=w987:T6)
              }
              frame "Exit" {
                # ">> State after true stop >>"
                # ">> Goes to true stop >>"
                n359 = for {
                  shift-right: [w1008] -> w1005
                  shift-left: w1002 -> [w1009]
                  tunnel: string[] ["STOP", "RESET ENCODERS", "RESET YAW", ""] -> [w1007] mode=indexing
                  n360 = Enqueue Element(queue=w1009, element=w1007) -> (queue out=w1008:refnum<queue>)  [unwired: 2 in, 2 out]
                }
              }
            }
          }
          frame 38 {
            # ">> Stepper height reeached >>"
            # ">>> yStepper command>>>"
            # ">> Manual override >>"
            n361 = Dequeue Element(queue=w1019, timeout in ms (-1)=w1014, error in (no error)=w1018) -> (element=w1022:T7)  [unwired: 3 out]
            n362 = Equal?(x=w1016, y=u8 80) -> (x = y?=w1020:bool)
            n363 = case shown="\"None\", Default" w1022 {
              tunnel: [w1033 State_Type_Definitions."True Stop" ("Enum")] -> w1012
              tunnel: [w1031 w1048] -> w1011
              tunnel: w1015 -> [w1030 _]
              tunnel: w1017 -> [w1024 _]
              tunnel: [State_Type_Definitions."Idle" ("Enum") State_Type_Definitions."Shutdown" ("Enum")] -> w1013
              tunnel: w1020 -> [w1023 _]
              frame "None", Default {
                # ">> WIill proceed to part ii if not manual override >>"
                # ">>If ENABLE or Trigger is set to true>>"
                n364 = Or(x=w1023, y=w1024) -> (x .or. y?=w1025:bool)
                n365 = case shown="True" w1023 {
                  tunnel: [w1036 w1042] -> w1031
                  tunnel: w1030 -> [w1035 w1041]
                  frame False {
                    n366 = for {
                      shift-right: [w1038] -> w1036
                      shift-left: w1035 -> [w1039]
                      tunnel: string[] ["Z STEPPER CAM HEIGHT", "READ STEPPER VALUES"] ("element") -> [w1037] mode=indexing
                      n367 = Enqueue Element(queue=w1039, element=w1037) -> (queue out=w1038:refnum<queue>)  [unwired: 2 in, 2 out]
                    }
                  }
                  frame True {
                    n368 = for {
                      shift-right: [w1044] -> w1042
                      shift-left: w1041 -> [w1045]
                      tunnel: string[] ["ARDUINO - ULTRASONIC", "READ ULTRASONIC", "", "", "", ""] -> [w1043] mode=indexing
                      n369 = Enqueue Element(queue=w1045, element=w1043) -> (queue out=w1044:refnum<queue>)  [unwired: 2 in, 2 out]
                    }
                  }
                }
                n370 = Select(t=State_Type_Definitions."True Stop" ("Enum"), s=w1024, f=State_Type_Definitions."Task 9B: Rotate to Angle" ("Enum")) -> (s? t:f=w1027:T6)
                n371 = Select(t=w1027, s=w1025, f=State_Type_Definitions."Task 9A: Raise Arm" ("Enum")) -> (s? t:f=w1033:T6)
              }
              frame "Exit" {
                n372 = for {
                  shift-right: [w1051] -> w1048
                  shift-left: _ -> [w1052]
                  tunnel: string[] ["STOP", "RESET ENCODERS", "RESET YAW", ""] -> [w1050] mode=indexing
                  n373 = Enqueue Element(queue=w1052, element=w1050) -> (queue out=w1051:refnum<queue>)  [unwired: 2 in, 2 out]
                }
              }
            }
          }
          frame 39 {
            # ">>> yStepper command>>>"
            n374 = Dequeue Element(queue=w1064, timeout in ms (-1)=w1063, error in (no error)=w1062) -> (element=w1066:T7)  [unwired: 3 out]
            n375 = In Range and Coerce(upper limit=305.0, x=w1056, lower limit=295.0) -> (In Range?=w1053:bool)  [unwired: 1 out]
            n376 = case shown="\"None\", Default" w1066 {
              tunnel: w1057 -> [w1069 _]
              tunnel: [w1077 State_Type_Definitions."True Stop" ("Enum")] -> w1059
              tunnel: w1065 -> [w1075 w1093]
              tunnel: [w1074 w1092] -> w1058
              tunnel: [State_Type_Definitions."Idle" ("Enum") State_Type_Definitions."Shutdown" ("Enum")] -> w1060
              tunnel: w1053 -> [w1067 _]
              frame "None", Default {
                n377 = Or(x=w1067, y=w1069) -> (x .or. y?=w1068:bool)
                n378 = case shown="True" w1067 {
                  tunnel: w1075 -> [w1080 w1086]
                  tunnel: [w1079 w1084] -> w1074
                  frame False {
                    n379 = for {
                      shift-right: [w1082] -> w1079
                      shift-left: w1080 -> [w1083]
                      tunnel: string[] ["READ NAVX", "R-ACW"] ("element") -> [w1081] mode=indexing
                      n380 = Enqueue Element(queue=w1083, element=w1081) -> (queue out=w1082:refnum<queue>)  [unwired: 2 in, 2 out]
                    }
                  }
                  frame True {
                    n381 = for {
                      shift-right: [w1088] -> w1084
                      shift-left: w1086 -> [w1089]
                      tunnel: string[] ["STOP", "RESET ENCODERS", "RESET YAW", ""] -> [w1087] mode=indexing
                      n382 = Enqueue Element(queue=w1089, element=w1087) -> (queue out=w1088:refnum<queue>)  [unwired: 2 in, 2 out]
                    }
                  }
                }
                n383 = Select(t=State_Type_Definitions."True Stop" ("Enum"), s=w1069, f=State_Type_Definitions."Task 9C: Rotation alignmnet") -> (s? t:f=w1071:u16)
                n384 = Select(t=w1071, s=w1068, f=State_Type_Definitions."Task 9B: Rotate to Angle" ("Enum")) -> (s? t:f=w1077:u16)
              }
              frame "Exit" {
                n385 = for {
                  shift-right: [w1096] -> w1092
                  shift-left: w1093 -> [w1097]
                  tunnel: string[] ["STOP", "RESET ENCODERS", "RESET YAW", ""] -> [w1095] mode=indexing
                  n386 = Enqueue Element(queue=w1097, element=w1095) -> (queue out=w1096:refnum<queue>)  [unwired: 2 in, 2 out]
                }
              }
            }
          }
          frame 33 {
            # ">>> yStepper command>>>"
            n387 = Dequeue Element(queue=w1106, timeout in ms (-1)=w1105, error in (no error)=w1104) -> (element=w1107:T7)  [unwired: 3 out]
            n388 = case shown="\"None\", Default" w1107 {
              tunnel: w1102 -> [w1108 _]
              tunnel: [w1116 State_Type_Definitions."True Stop" ("Enum")] -> w1099
              tunnel: w1103 -> [w1114 w1132]
              tunnel: [w1113 w1131] -> w1098
              tunnel: [State_Type_Definitions."Idle" ("Enum") State_Type_Definitions."Shutdown" ("Enum")] -> w1101
              frame "None", Default {
                n389 = case shown="True" w1108 {
                  tunnel: w1114 -> [w1119 w1125]
                  tunnel: [w1118 w1123] -> w1113
                  frame False {
                    n390 = for {
                      shift-right: [w1121] -> w1118
                      shift-left: w1119 -> [w1122]
                      tunnel: string[] ["READ IR", "FORWARD - IR ASSIST"] ("element") -> [w1120] mode=indexing
                      n391 = Enqueue Element(queue=w1122, element=w1120) -> (queue out=w1121:refnum<queue>)  [unwired: 2 in, 2 out]
                    }
                  }
                  frame True {
                    n392 = for {
                      shift-right: [w1127] -> w1123
                      shift-left: w1125 -> [w1128]
                      tunnel: string[] ["STOP", "RESET ENCODERS", "RESET YAW", ""] -> [w1126] mode=indexing
                      n393 = Enqueue Element(queue=w1128, element=w1126) -> (queue out=w1127:refnum<queue>)  [unwired: 2 in, 2 out]
                    }
                  }
                }
                n394 = Select(t=State_Type_Definitions."True Stop" ("Enum"), s=w1108, f=State_Type_Definitions."True Stop") -> (s? t:f=w1110:T6)
                n395 = Select(t=w1110, s=w1108, f=State_Type_Definitions."Task 9C: Rotation alignmnet" ("Enum")) -> (s? t:f=w1116:u16)
              }
              frame "Exit" {
                n396 = for {
                  shift-right: [w1135] -> w1131
                  shift-left: w1132 -> [w1136]
                  tunnel: string[] ["STOP", "RESET ENCODERS", "RESET YAW", ""] -> [w1134] mode=indexing
                  n397 = Enqueue Element(queue=w1136, element=w1134) -> (queue out=w1135:refnum<queue>)  [unwired: 2 in, 2 out]
                }
              }
            }
          }
        }
      }
    }
    n398 = local write "Green LED"(w199) -> ()
  }
  n399 = call <vilib>:"DIO Close.vi"("error in (no error)"=w25, "DIO Info In"=w28) -> ()  [unwired: 9 in, 1 out]
  n400 = call <vilib>:"DIO Close.vi"("error in (no error)"=w35, "DIO Info In"=w37) -> ()  [unwired: 9 in, 1 out]
  n401 = call <vilib>:"NavX Close.vi"("error in (no error)"=w6, "NavX Info In"=w5) -> ()  [unwired: 9 in, 1 out]
  n402 = call <vilib>:"DIO Close.vi"("error in (no error)"=w30, "DIO Info In"=w32) -> ()  [unwired: 9 in, 1 out]
  n403 = call <vilib>:"DIO Close.vi"("error in (no error)"=w13, "DIO Info In"=w14) -> ()  [unwired: 9 in, 1 out]
  n404 = call <vilib>:"DIO Close.vi"("error in (no error)"=w8, "DIO Info In"=w9) -> ()  [unwired: 9 in, 1 out]
  n405 = while {
    stop <- w1636 stop-if-true
    n406 = call <vilib>:"RT Get CPU Loads.vi"() -> ("CPU loads"=→"CPU loads":T5[])  [unwired: 10 in, 1 out]
    n407 = Wait (ms)(milliseconds to wait=u32 100) -> ()  [unwired: 1 out]
    n408 = call "FGV Bool.vi"("Init/Read/Write State"=States_for_Action_Engine."Read") -> ("Output node"=w1636:bool)  [unwired: 2 in, 1 out]
  }
  n409 = while {
    stop <- w1640 stop-if-true
    n410 = call "MOTOR CONTROL WITH PID AE.vi"("AE Mode"=MOTOR_CONTROL_WITH_PID_AE_DATA_MODE_TYPE_DEF."Read from AE") -> ("Speed & distance"=→"Speed & distance":T1)  [unwired: 3 in]
    n411 = call "FGV Bool.vi"("Init/Read/Write State"=States_for_Action_Engine."Read") -> ("Output node"=w1640:bool)  [unwired: 2 in, 1 out]
    n412 = Wait (ms)(milliseconds to wait=u32 5) -> ()  [unwired: 1 out]
  }
  n413 = Merge Errors "Merge Errors"(w65, w64) -> (w47:errorcluster)
  n414 = Merge Errors(w51, w47) -> (w46:errorcluster)
  n415 = Destroy User Event(user event=w68, error in=w46) -> ()  [unwired: 1 out]
  n416 = Destroy User Event(user event=w69, error in=w46) -> ()  [unwired: 1 out]
  n417 = Unregister For Events(event registration refnum=w60, error in=w46) -> ()  [unwired: 1 out]
  n418 = Release Queue(queue=w42, error in (no error)=w46) -> (error out=w24:errorcluster)  [unwired: 1 in, 2 out]
  n419 = Release Queue(queue=w59, error in (no error)=w46) -> ()  [unwired: 1 in, 3 out]
  n420 = call <vilib>:"Simple Error Handler.vi"("error in (no error)"=w24) -> ("error out"=w23:errorcluster)  [unwired: 4 in, 4 out]
  n421 = call <vilib>:"Reset myRIO.vi"("error in (no error)"=w23) -> ("error out"=→"error out":errorcluster)  [unwired: 10 in]
